vi "main.vi"() -> ()   [LabVIEW 2015]
uses:
  C:/Users/tosun_2/Desktop/Interop.TSMasterAPI.dll
panel:
  in  "停止":bool
  in  "close":bool
  out "log":string
  in  "main tab":enum32{"启动", "数据库", "收发界面"}(tab)
  in  "使能flexray通道数量":i32
  in  "LIN通道配置":T1(array[cluster]) {"AFunctionType" items=["T_MasterNode", "T_SlaveNode", "T_MonitorNode"]; "AProtocol" items=["LIN_PROTOCOL_13", "LIN_PROTOCOL_20", "LIN_PROTOCOL_21", "LIN_PROTOCOL_J2602"]; "FHWDeviceSubType" items=["TS_UNKNOWN_DEVICE"=0, "TC1001 "=3, "TL1001"=4, "TC1011"=5, "TC1002"=7, "TC1014"=8, "TC1026"=10, "TC1016"=11, "TC1012"=12, "TC1013 "=13, "TC1034"=15]; "FHWDeviceType" items=["BUS_UNKNOWN_TYPE", "TS_TCP_DEVICE", "XL_USB_DEVICE", "TS_USB_DEVICE", "PEAK_USB_DEVICE", "KVASER_USB_DEVICE", "RESERVED_DEVICE", "ICS_USB_DEVICE", "TS_TC1005_DEVICE"]; "FHWChannelIndex" items=["CHN1", "CHN2", "CHN3", "CHN4", "CHN5", "CHN6", "CHN7", "CHN8", "CHN9", "CHN10", "CHN11", "CHN12", "CHN13", "CHN14", "CHN15", "CHN16", "CHN17", "CHN18", "CHN19", "CHN20", "CHN21", "CHN22", "CHN23", "CHN24", "CHN25", "CHN26", "CHN27", "CHN28", "CHN29", "CHN30", "CHN31", "CHN32"]}
  in  "connect":bool
  in  "open":bool
  in  "TSMaster工程路径（可选）":path
  in  "使能CAN通道数量":i32
  in  "dbc路径":path
  in  "CAN通道配置":T2(array[cluster]) {"FHWDeviceSubType" items=["TS_UNKNOWN_DEVICE"=0, "TC1001 "=3, "TL1001"=4, "TC1011"=5, "TC1002"=7, "TC1014"=8, "TC1026"=10, "TC1016"=11, "TC1012"=12, "TC1013 "=13, "TC1034"=15]; "AControllerMode" items=["lfdmNormal", "lfdmACKOff", "lfdmRestricted"]; "AControllerType" items=["lfdtCAN", "lfdtISOFDCAN", "lfdtNonISOFDFDCAN"]; "FHWDeviceType" items=["BUS_UNKNOWN_TYPE", "TS_TCP_DEVICE", "XL_USB_DEVICE", "TS_USB_DEVICE", "PEAK_USB_DEVICE", "KVASER_USB_DEVICE", "RESERVED_DEVICE", "ICS_USB_DEVICE", "TS_TC1005_DEVICE"]; "FHWChannelIndex" items=["CHN1", "CHN2", "CHN3", "CHN4", "CHN5", "CHN6", "CHN7", "CHN8", "CHN9", "CHN10", "CHN11", "CHN12", "CHN13", "CHN14", "CHN15", "CHN16", "CHN17", "CHN18", "CHN19", "CHN20", "CHN21", "CHN22", "CHN23", "CHN24", "CHN25", "CHN26", "CHN27", "CHN28", "CHN29", "CHN30", "CHN31", "CHN32"]}
  in  "使能LIN通道数量":i32
  in  "ldf路径":path
  in  "xml路径":path
  in  "refresh databases":bool
  in  "数据库选项卡":enum32{"CAN", "LIN", "flexray"}(tab)
  out "CAN database":string(tree)="_1"
  out "LIN database":string(tree)="_1" caption="CAN database"
  out "flexray database":string(tree)="_1" caption="CAN database"
  in  "transmit":bool
  in  "transtab":enum32{"CAN", "LIN", "flexray"}(tab)
  in  "CAN通道":u8
  in  "CAN ID":i32 format="%x"
  in  "是否远程帧":bool
  in  "是否扩展帧":bool
  in  "是否CAN FD":bool
  in  "是否BRS":bool
  in  "DLC":u8
  in  "数据":u8[](array[numeric])
  in  "LIN通道":u8
  in  "LIN ID":u8 format="%x"
  in  "长度":u8
  in  "数据":u8[](array[numeric])
  in  "是否包含数据":bool=TRUE
  in  "数据 2":u8[](array[numeric])
  in  "flexray通道":u8
  in  "SlotId":u16
  in  "CycleNumber":u8
  in  "负载长度":u8
  in  "报文信息":i32(listbox)
  # "做主节点，不使能发送的flag时：设备将发送LIN报头，借此像从节点请求数据。做从节点时，仅更新数据，不会主动发送。"
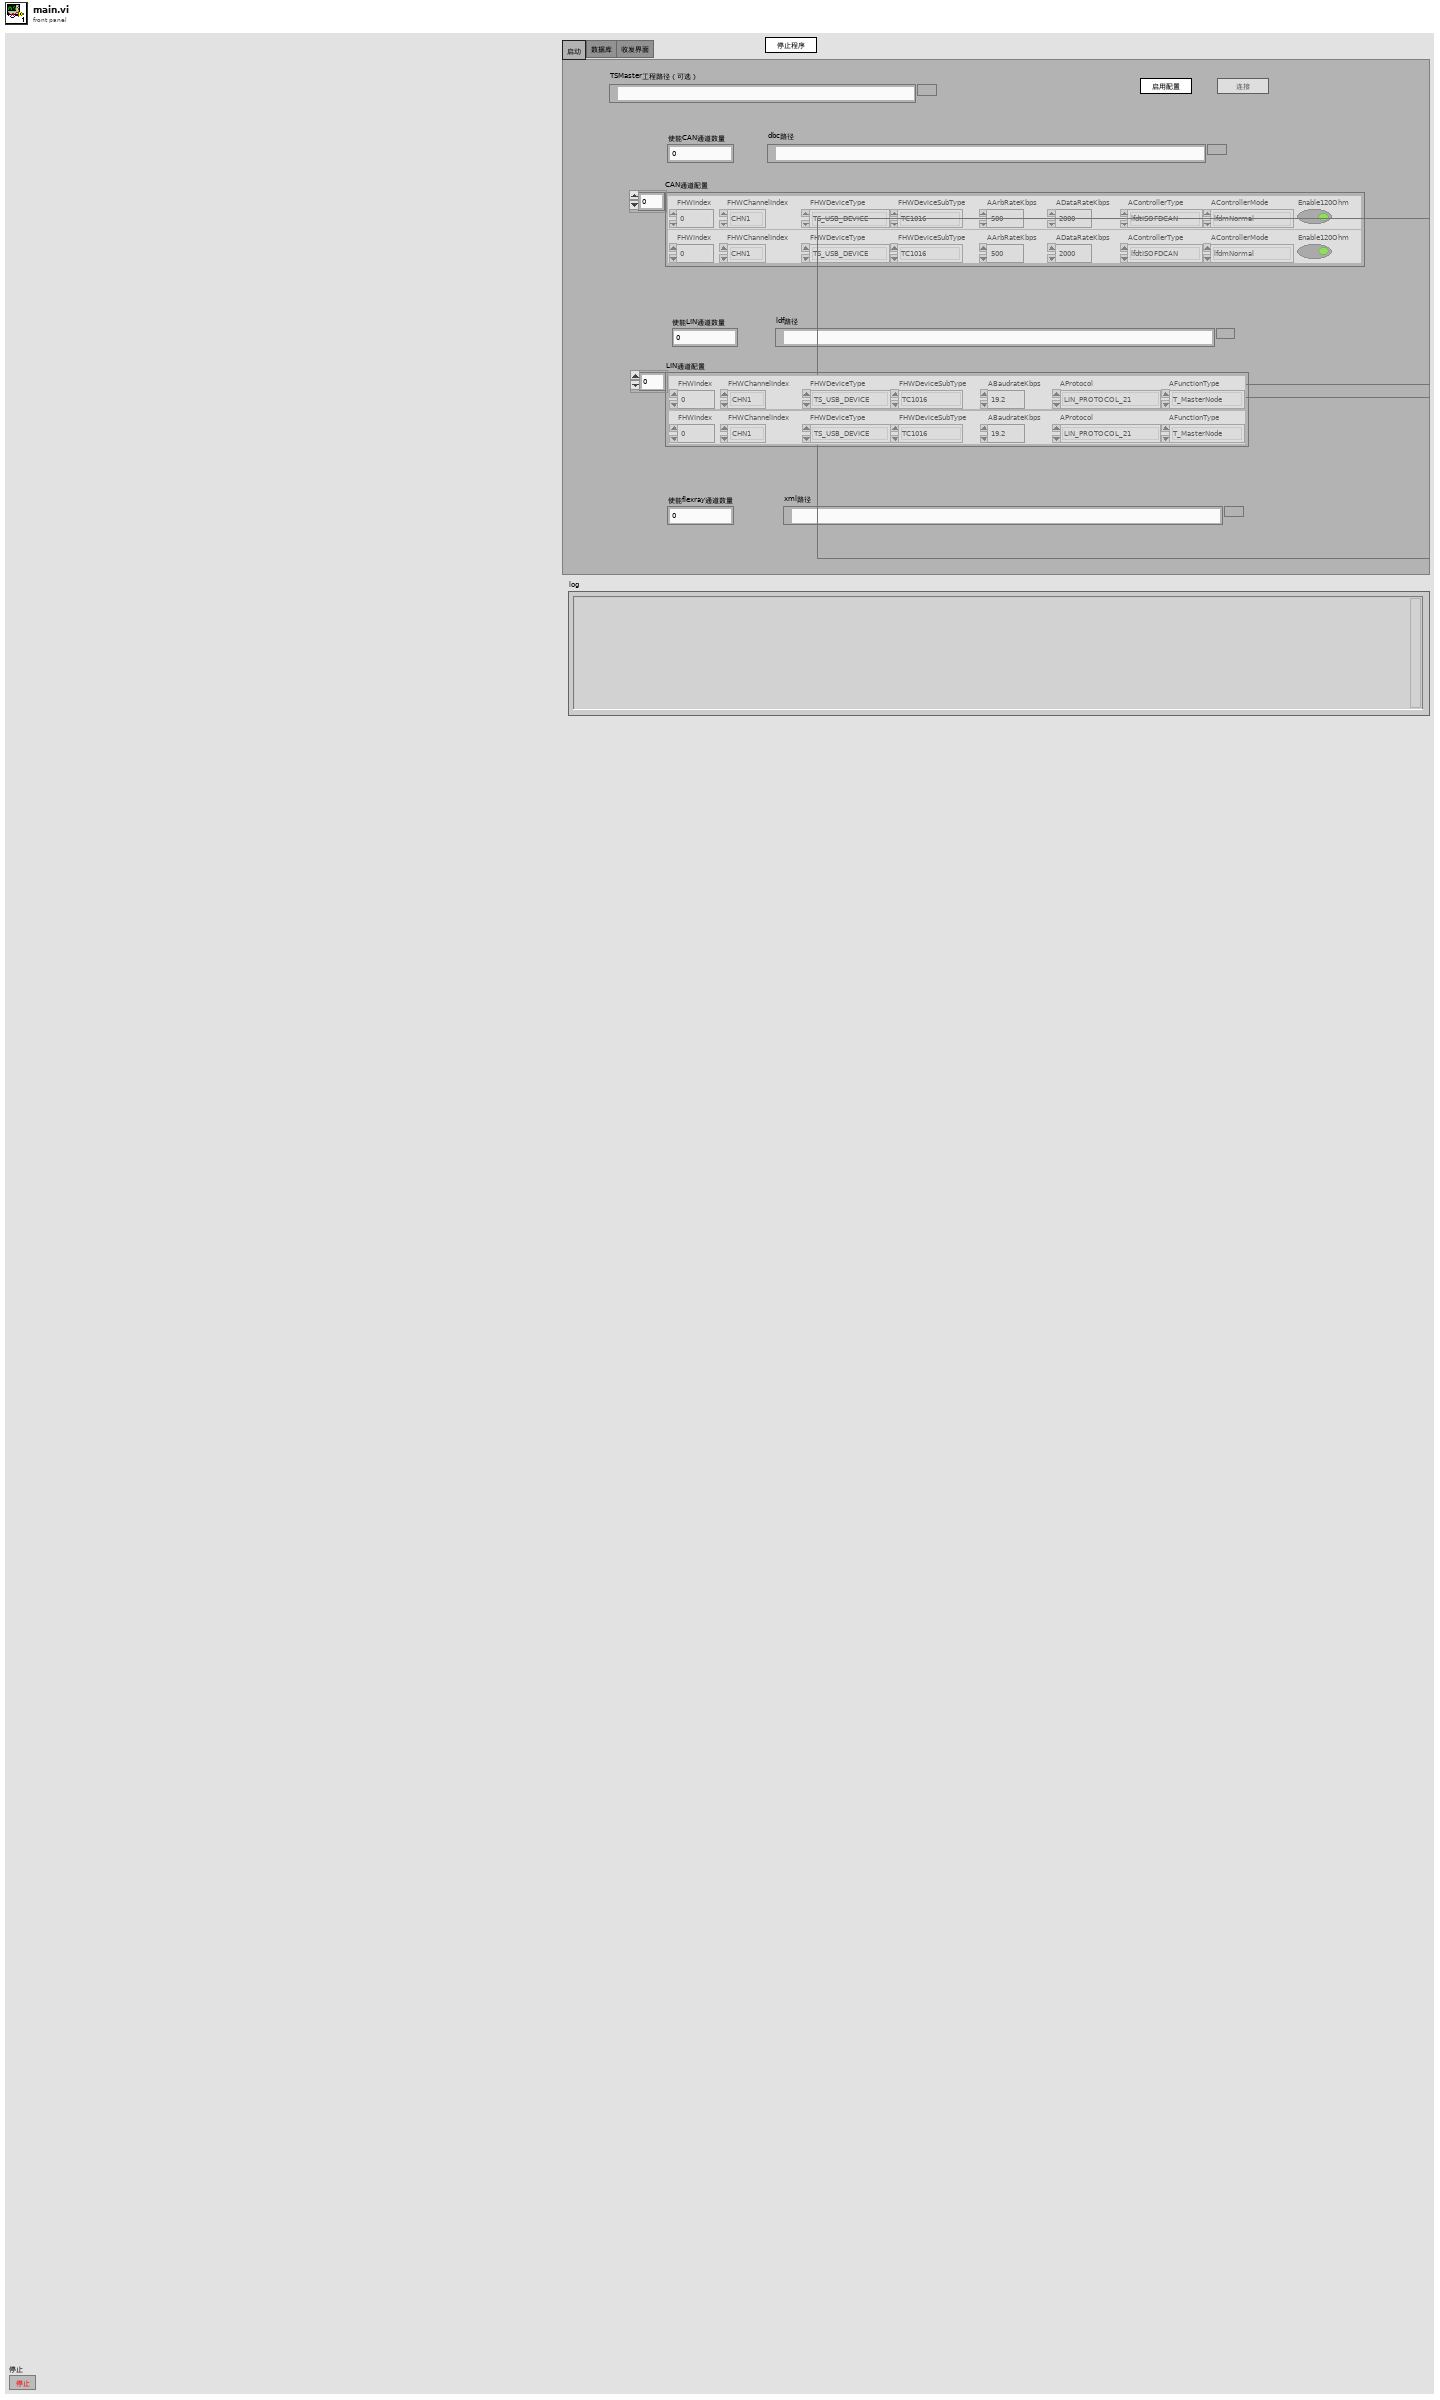
[diagram p1: front panel]
types:
  T1 = cluster{"FHWIndex":i32, "FHWChannelIndex":i32, "FHWDeviceType":i32, "FHWDeviceSubType":i32, "ABaudrateKbps":sgl, "AProtocol":i32, "AFunctionType":i32}[]
  T2 = cluster{"FHWIndex":i32, "FHWChannelIndex":i32, "FHWDeviceType":i32, "FHWDeviceSubType":i32, "AArbRateKbps":sgl, "ADataRateKbps":sgl, "AControllerType":i32, "AControllerMode":i32, "Enable120Ohm":bool}[]
  T3 = enum8{"Enabled", "Disabled", "Disabled and Grayed Out"}
  T4 = cluster{"Left Cell String":string, "Child Text":string[], "Child Tag":string, "Item Indent":i32, "Child Only?":bool, "Glyph Index":i32}[]
  T5 = cluster{"Left Cell String":string, "Child Text":string[], "Child Tag":string, "Item Indent":i32, "Child Only?":bool, "Glyph Index":i32}
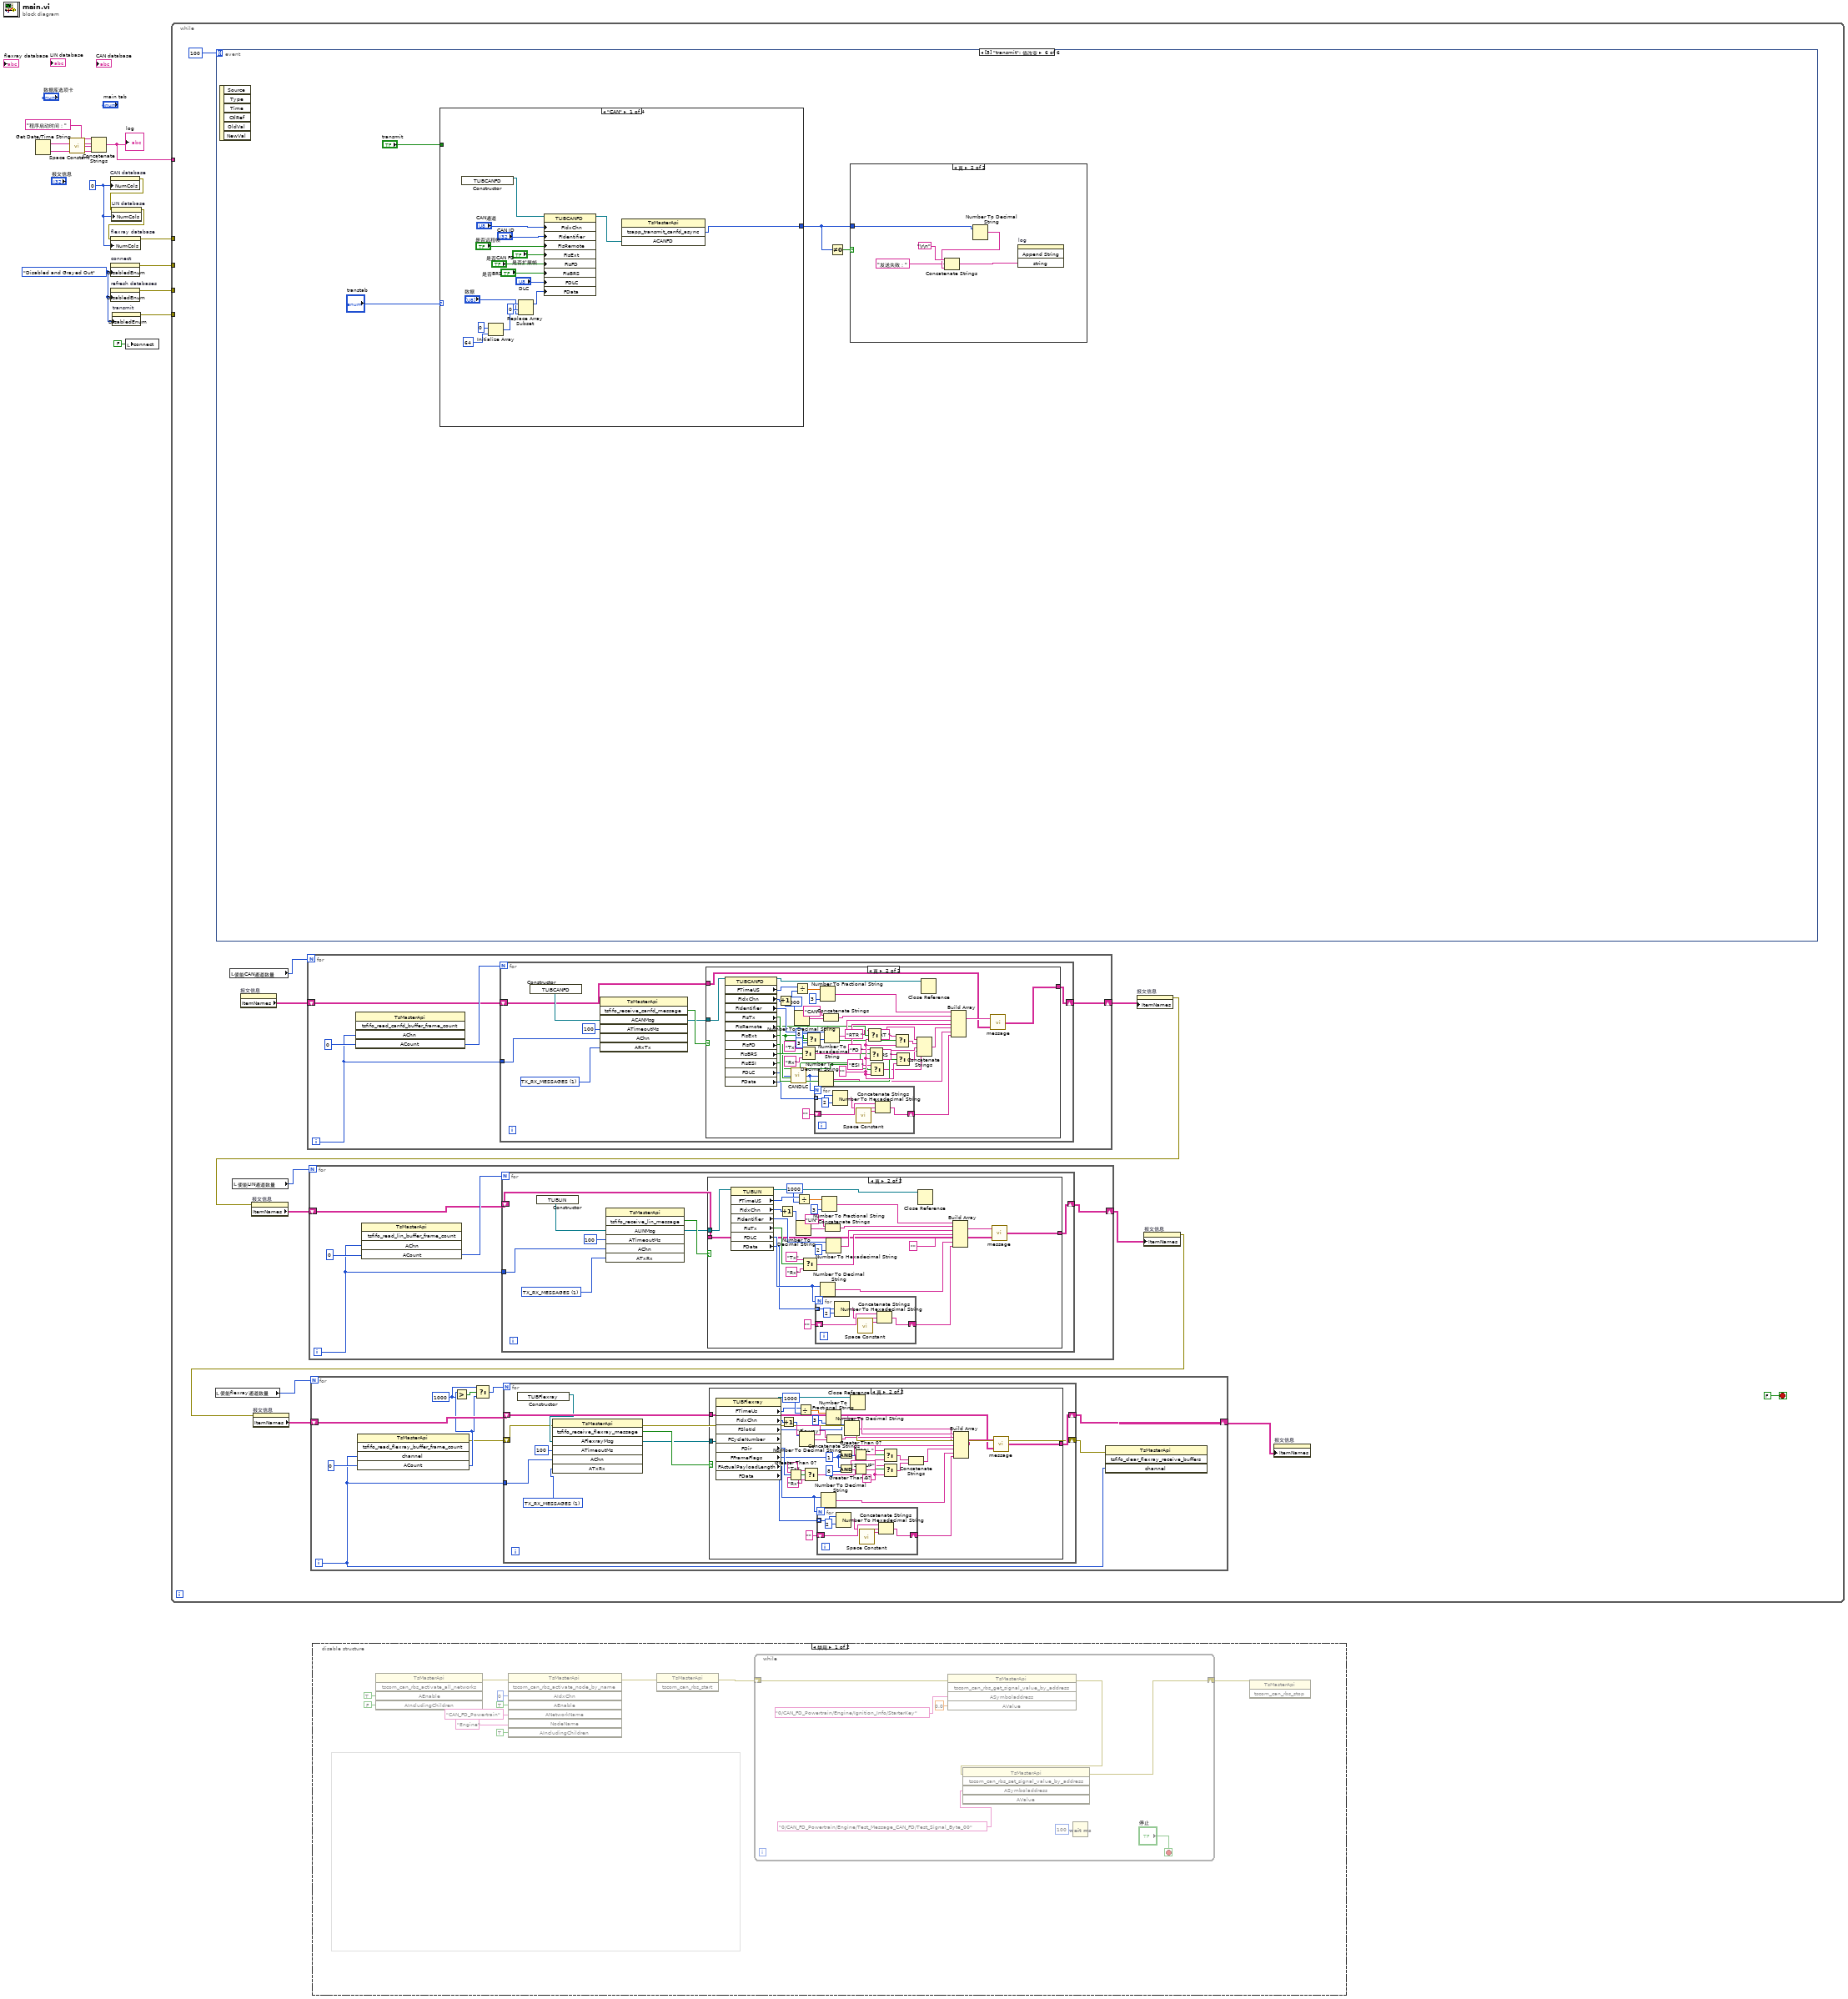
[diagram p0: block diagram]
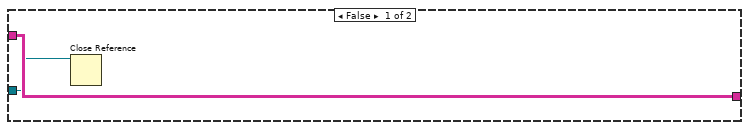
[diagram p3: hidden frame]
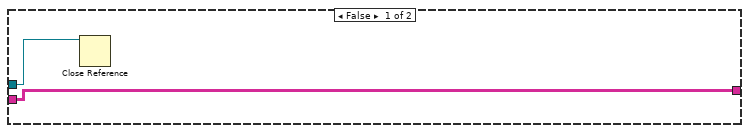
[diagram p4: hidden frame]
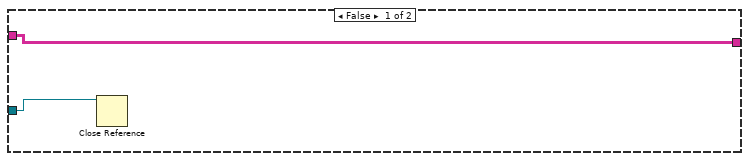
[diagram p5: hidden frame]
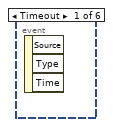
[diagram p6: hidden frame]
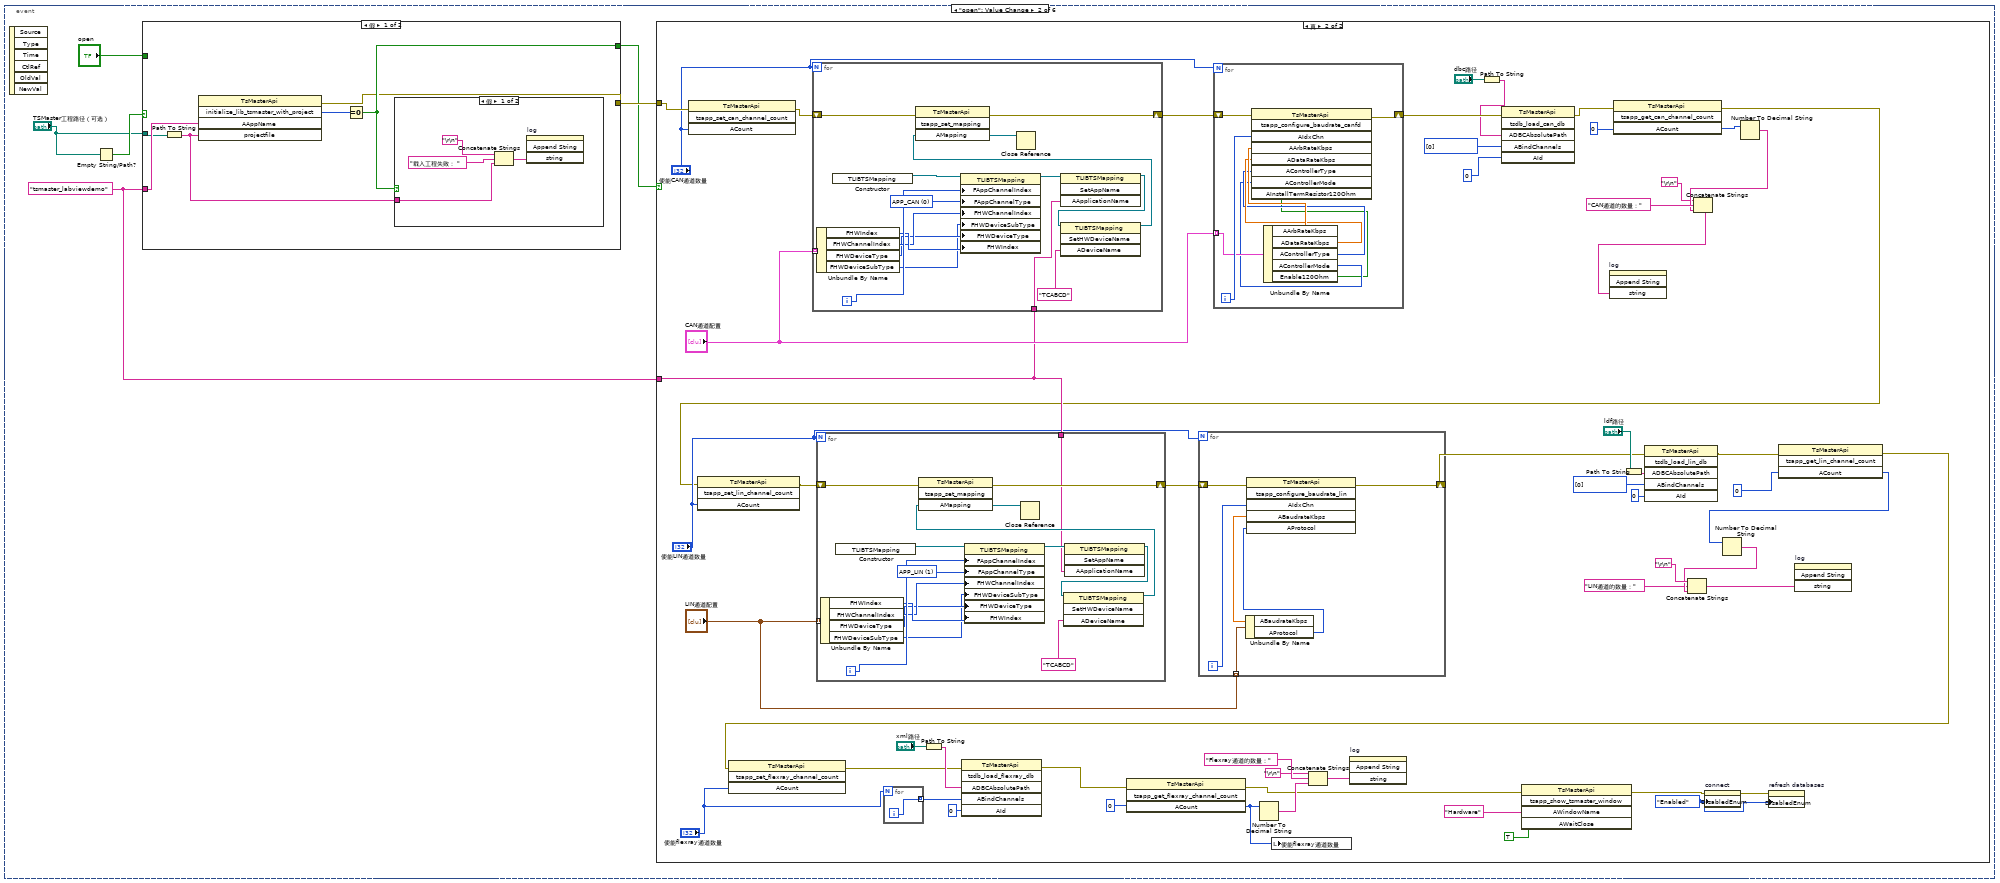
[diagram p7: hidden frame]
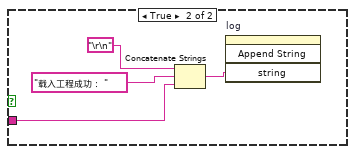
[diagram p9: hidden frame]
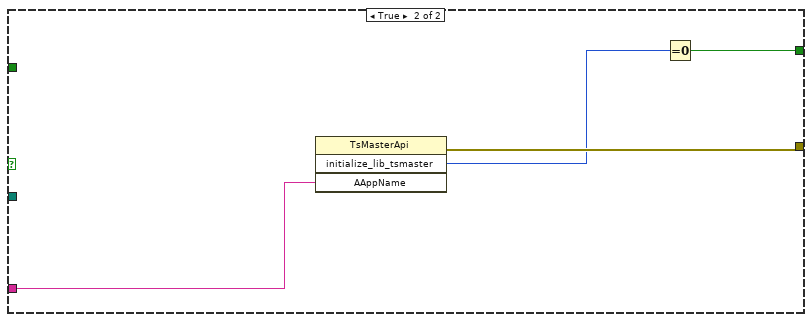
[diagram p10: hidden frame]
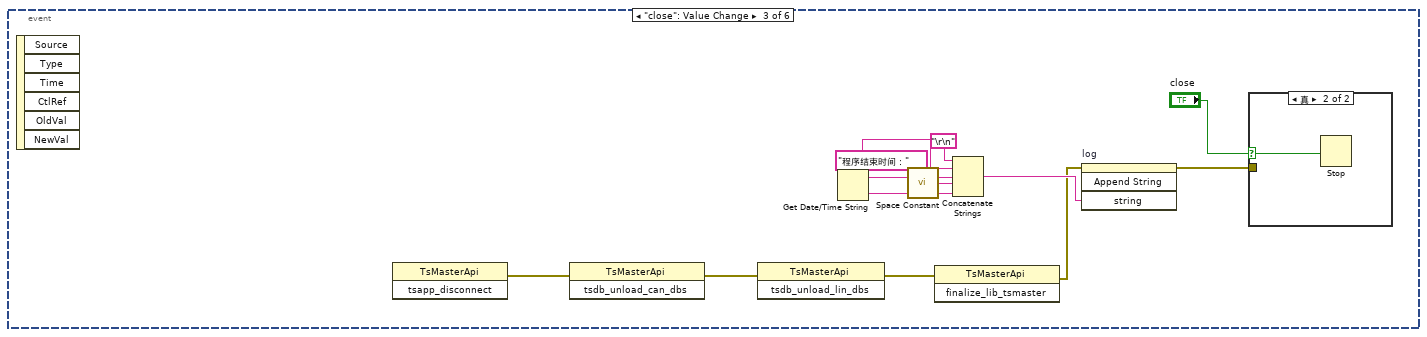
[diagram p11: hidden frame]
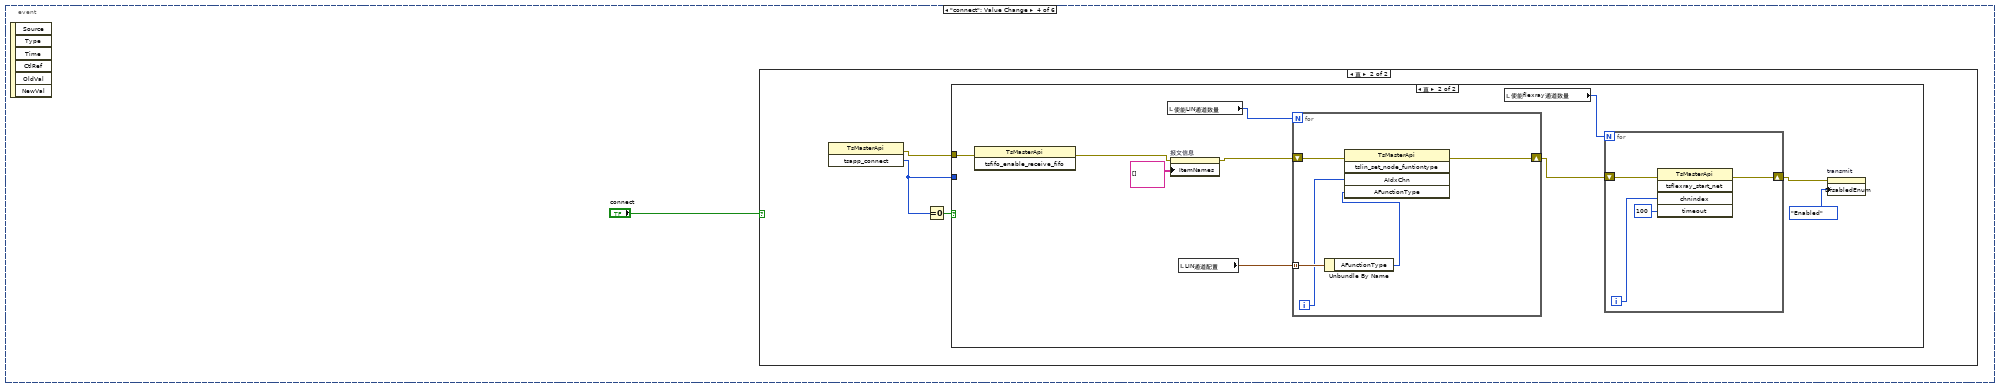
[diagram p13: hidden frame]
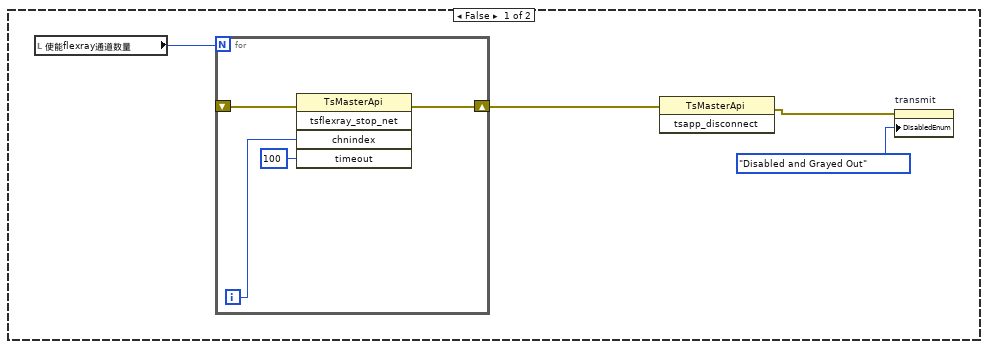
[diagram p14: hidden frame]
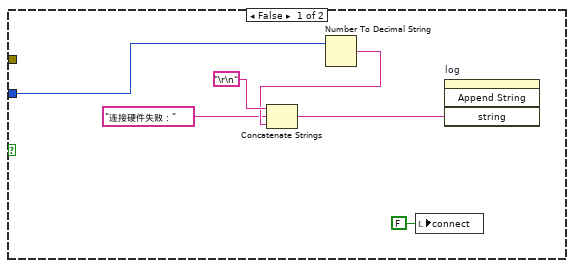
[diagram p15: hidden frame]
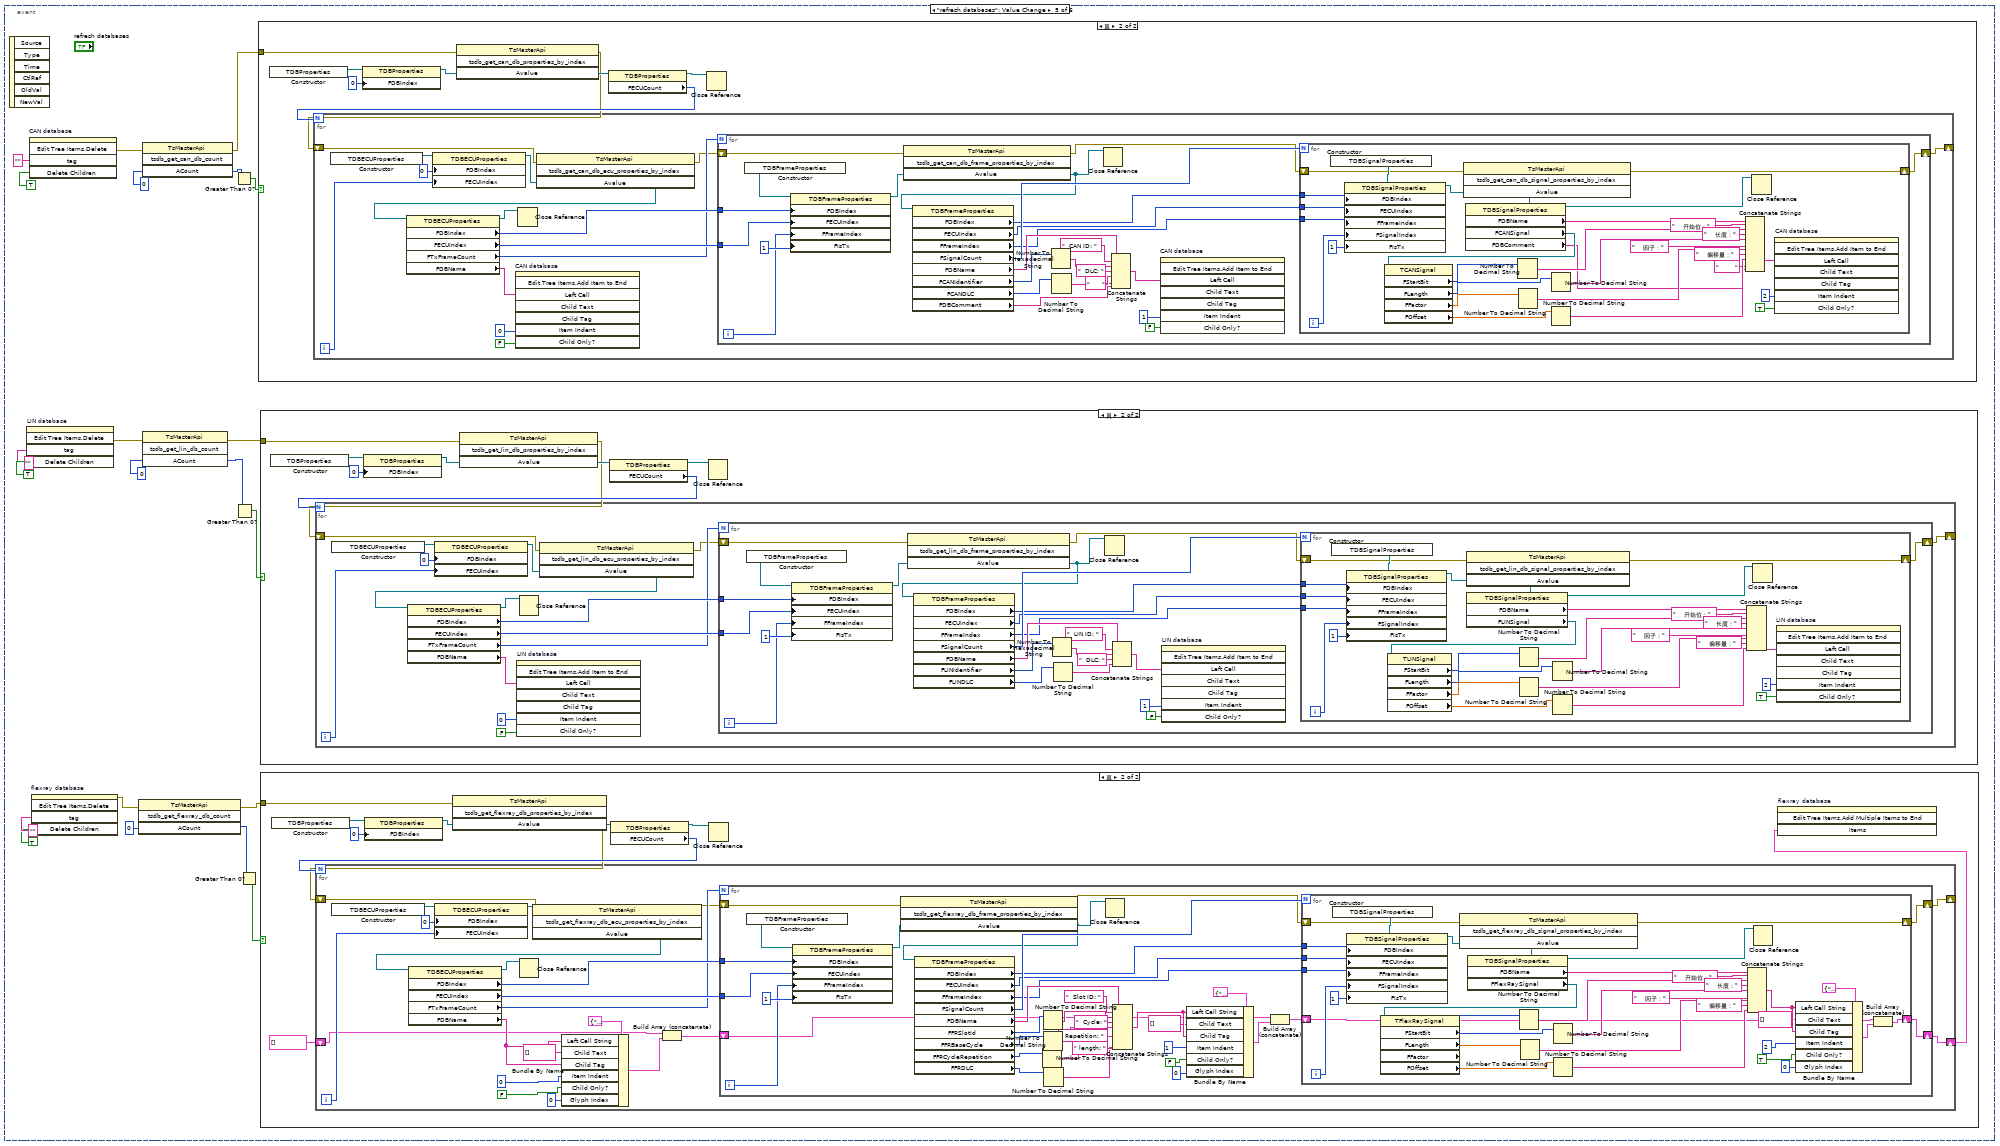
[diagram p16: hidden frame]
diagram:
  w3 = T3."Disabled and Grayed Out" ("禁用")
  w6 = u32 0 ("列数")
  n1 = Get Date/Time String() -> (date string=w13:string, time string=w12:string)  [unwired: 3 in]
  n2 = call <vilib>:"Space Constant.vi"() -> ("String"=w10:string)
  n3 = Concatenate Strings("程序启动时间：" ("字符串"), w13, w10, w12) -> (w11:string)
  "log" <- w11
  n4 = property on="CAN database" class="Tree (严格)"("NumCols"=w6) -> (error out=w9:errorcluster)  [unwired: 2 in, 1 out]
  n5 = property on="connect" class="Bool (严格)"("DisabledEnum"=w3) -> (error out=w5:errorcluster)  [unwired: 2 in, 1 out]
  n6 = property on="refresh databases" class="Bool"("DisabledEnum"=w3) -> (error out=w4:errorcluster)  [unwired: 2 in, 1 out]
  n7 = property on="LIN database" class="Tree (严格)"(error in=w9, "NumCols"=w6) -> (error out=w7:errorcluster)  [unwired: 1 in, 1 out]
  n8 = property on="flexray database" class="Tree (严格)"(error in=w7, "NumCols"=w6) -> (error out=w8:errorcluster)  [unwired: 1 in, 1 out]
  n9 = property on="transmit" class="Bool"("DisabledEnum"=w3) -> (error out=w2:errorcluster)  [unwired: 2 in, 1 out]
  n10 = local write "connect"(FALSE ("connect")) -> ()
  n11 = while {
    tunnel: w11 -> [_]
    tunnel: w8 -> [_]
    tunnel: w5 -> [_]
    tunnel: w4 -> [_]
    tunnel: w2 -> [_]
    stop <- FALSE stop-if-true
    n12 = local read "使能flexray通道数量"() -> (w17:i32)
    n13 = event shown="[5] \"transmit\": 值改变" {
      selector: _ -> [_ _ _ _ _ _]
      dyn-events: _ -> [_ _ _ _ _ _]
      timeout: 100 -> [_ _ _ _ _ _]
      event Timeout {
        n14 = event-data() -> ()  [unwired: 1 in, 3 out]
      }
      event "open": Value Change {
        w213 = "tsmaster_labviewdemo" ("AAppName")
        n15 = event-data() -> ()  [unwired: 1 in, 6 out]
        n16 = Empty String/Path?(string/path="TSMaster工程路径（可选）") -> (empty?=w218:bool)
        n17 = case shown="假" w218 {
          tunnel: "open" -> [_ _]
          tunnel: w213 -> [w327 w339]
          tunnel: "TSMaster工程路径（可选）" -> [w326 _]
          tunnel: [w324 w338] -> w214
          tunnel: [w322 w337] -> w215
          frame False {
            n18 = Path To String(path=w326) -> (string=w323:string)
            n19 = invoke on="调用节点" class="TsMasterApi" method="initialize_lib_tsmaster_with_project"("AAppName"=w327, "projectfile"=w323) -> (error out=w322:errorcluster, "initialize_lib_tsmaster_with_project"=w325:i32)  [unwired: 3 in, 3 out]
            n20 = Equal To 0?(x=w325) -> (x = 0?=w324:bool)
            n21 = case shown="假" w324 {
              tunnel: w323 -> [w329 w332]
              frame False {
                n22 = Concatenate Strings("\r\n", "载入工程失败： " ("字符串"), w329) -> (w328:string)
                n23 = invoke on="log" class="Str" method="Append String"("string"=w328) -> ()  [unwired: 3 in, 4 out]
              }
              frame True {
                n24 = Concatenate Strings("\r\n", "载入工程成功： " ("字符串"), w332) -> (w335:string)
                n25 = invoke on="log" class="Str" method="Append String"("string"=w335) -> ()  [unwired: 3 in, 4 out]
              }
            }
          }
          frame True {
            n26 = invoke on="调用节点" class="TsMasterApi" method="initialize_lib_tsmaster"("AAppName"=w339) -> (error out=w337:errorcluster, "initialize_lib_tsmaster"=w336:i32)  [unwired: 3 in, 2 out]
            n27 = Equal To 0?(x=w336) -> (x = 0?=w338:bool)
          }
        }
        n28 = case shown="真" w214 {
          tunnel: w215 -> [_ w261]
          tunnel: w213 -> [_ w256]
          frame False {
          }
          frame True {
            w221 = T3."Enabled" ("禁用")
            w250 = i32[] [0] items=["CHN1", "CHN2", "CHN3", "CHN4", "CHN5", "CHN6", "CHN7", "CHN8", "CHN9", "CHN10", "CHN11", "CHN12", "CHN13", "CHN14", "CHN15", "CHN16", "CHN17", "CHN18", "CHN19", "CHN20", "CHN21", "CHN22", "CHN23", "CHN24", "CHN25", "CHN26", "CHN27", "CHN28", "CHN29", "CHN30", "CHN31", "CHN32"] ("ABindChannels")
            w263 = i32[] [0] items=["CHN1", "CHN2", "CHN3", "CHN4", "CHN5", "CHN6", "CHN7", "CHN8", "CHN9", "CHN10", "CHN11", "CHN12", "CHN13", "CHN14", "CHN15", "CHN16", "CHN17", "CHN18", "CHN19", "CHN20", "CHN21", "CHN22", "CHN23", "CHN24", "CHN25", "CHN26", "CHN27", "CHN28", "CHN29", "CHN30", "CHN31", "CHN32"] ("ABindChannels")
            n29 = invoke on="调用节点" class="TsMasterApi" method="tsapp_set_can_channel_count"(error in=w261, "ACount"="使能CAN通道数量") -> (error out=w260:errorcluster)  [unwired: 2 in, 3 out]
            n30 = for {
              N: "使能CAN通道数量" -> [_]
              shift-right: [w321] -> w239
              shift-left: w260 -> [w314]
              tunnel: "CAN通道配置" -> [w318] mode=indexing
              tunnel: w256 -> [w308]
              i -> [w319]
              w320 = 0 items=["APP_CAN", "APP_LIN"] ("FAppChannelType")
              n31 = Unbundle By Name(w318) -> ("FHWIndex"=w317:i32, "FHWChannelIndex"=w316:i32, "FHWDeviceType"=w315:i32, "FHWDeviceSubType"=w306:i32)
              n32 = constructor class="TLIBTSMapping"() -> (reference out=w313:refnum<k24>)  [unwired: 3 in, 2 out]
              n33 = property on="属性节点" class="TLIBTSMapping"(reference=w313, "FAppChannelIndex"=w319, "FAppChannelType"=w320, "FHWChannelIndex"=w316, "FHWDeviceSubType"=w306, "FHWDeviceType"=w315, "FHWIndex"=w317) -> (reference out=w312:refnum<k24>)  [unwired: 1 in, 1 out]
              n34 = invoke on="调用节点" class="TLIBTSMapping" method="SetAppName"(reference=w312, "AApplicationName"=w308) -> (reference out=w310:refnum<k24>)  [unwired: 2 in, 3 out]
              n35 = invoke on="调用节点" class="TLIBTSMapping" method="SetHWDeviceName"(reference=w310, "ADeviceName"="TCABCD") -> (reference out=w309:refnum<k24>)  [unwired: 2 in, 3 out]
              n36 = invoke on="调用节点" class="TsMasterApi" method="tsapp_set_mapping"(error in=w314, "AMapping"=w309) -> (error out=w321:errorcluster, "AMapping"=w307:refnum<k24>)  [unwired: 2 in, 2 out]
              n37 = Close Reference(reference=w307) -> ()  [unwired: 1 in, 1 out]
            }
            n38 = for {
              N: "使能flexray通道数量" -> [_]
              tunnel: [w274] -> w224 mode=indexing
              i -> [w274]
            }
            n39 = Path To String(path="xml路径") -> (string=w227:string)
            n40 = for {
              N: "使能CAN通道数量" -> [_]
              shift-right: [w304] -> w266
              shift-left: w239 -> [w305]
              tunnel: "CAN通道配置" -> [w302] mode=indexing
              i -> [w303]
              n41 = Unbundle By Name(w302) -> ("AArbRateKbps"=w301:sgl, "ADataRateKbps"=w300:sgl, "AControllerType"=w299:i32, "AControllerMode"=w298:i32, "Enable120Ohm"=w297:bool)
              n42 = invoke on="调用节点" class="TsMasterApi" method="tsapp_configure_baudrate_canfd"(error in=w305, "AIdxChn"=w303, "AArbRateKbps"=w301, "ADataRateKbps"=w300, "AControllerType"=w299, "AControllerMode"=w298, "AInstallTermResistor120Ohm"=w297) -> (error out=w304:errorcluster)  [unwired: 2 in, 8 out]
            }
            n43 = Path To String(path="dbc路径") -> (string=w264:string)
            n44 = invoke on="调用节点" class="TsMasterApi" method="tsdb_load_can_db"(error in=w266, "ADBCAbsolutePath"=w264, "ABindChannels"=w263, "AId"=u32 0) -> (error out=w259:errorcluster)  [unwired: 2 in, 5 out]
            n45 = invoke on="调用节点" class="TsMasterApi" method="tsapp_get_can_channel_count"(error in=w259, "ACount"=0) -> (error out=w253:errorcluster, "ACount"=w268:i32)  [unwired: 2 in, 2 out]
            n46 = invoke on="调用节点" class="TsMasterApi" method="tsapp_set_lin_channel_count"(error in=w253, "ACount"="使能LIN通道数量") -> (error out=w257:errorcluster)  [unwired: 2 in, 3 out]
            n47 = for {
              N: "使能LIN通道数量" -> [_]
              shift-right: [w296] -> w240
              shift-left: w257 -> [w289]
              tunnel: "LIN通道配置" -> [w293] mode=indexing
              tunnel: w256 -> [w281]
              i -> [w294]
              w295 = 1 items=["APP_CAN", "APP_LIN"] ("FAppChannelType")
              n48 = Unbundle By Name(w293) -> ("FHWIndex"=w292:i32, "FHWChannelIndex"=w291:i32, "FHWDeviceType"=w290:i32, "FHWDeviceSubType"=w282:i32)
              n49 = constructor class="TLIBTSMapping"() -> (reference out=w288:refnum<k24>)  [unwired: 3 in, 2 out]
              n50 = property on="属性节点" class="TLIBTSMapping"(reference=w288, "FAppChannelIndex"=w294, "FAppChannelType"=w295, "FHWChannelIndex"=w291, "FHWDeviceSubType"=w282, "FHWDeviceType"=w290, "FHWIndex"=w292) -> (reference out=w287:refnum<k24>)  [unwired: 1 in, 1 out]
              n51 = invoke on="调用节点" class="TLIBTSMapping" method="SetAppName"(reference=w287, "AApplicationName"=w281) -> (reference out=w285:refnum<k24>)  [unwired: 2 in, 3 out]
              n52 = invoke on="调用节点" class="TLIBTSMapping" method="SetHWDeviceName"(reference=w285, "ADeviceName"="TCABCD") -> (reference out=w284:refnum<k24>)  [unwired: 2 in, 3 out]
              n53 = invoke on="调用节点" class="TsMasterApi" method="tsapp_set_mapping"(error in=w289, "AMapping"=w284) -> (error out=w296:errorcluster, "AMapping"=w283:refnum<k24>)  [unwired: 2 in, 2 out]
              n54 = Close Reference(reference=w283) -> ()  [unwired: 1 in, 1 out]
            }
            n55 = for {
              N: "使能LIN通道数量" -> [_]
              shift-right: [w275] -> w241
              shift-left: w240 -> [w280]
              tunnel: "LIN通道配置" -> [w279] mode=indexing
              i -> [w276]
              n56 = Unbundle By Name(w279) -> ("ABaudrateKbps"=w278:sgl, "AProtocol"=w277:i32)
              n57 = invoke on="调用节点" class="TsMasterApi" method="tsapp_configure_baudrate_lin"(error in=w280, "AIdxChn"=w276, "ABaudrateKbps"=w278, "AProtocol"=w277) -> (error out=w275:errorcluster)  [unwired: 2 in, 5 out]
            }
            n58 = Path To String(path="ldf路径") -> (string=w249:string)
            n59 = invoke on="调用节点" class="TsMasterApi" method="tsdb_load_lin_db"(error in=w241, "ADBCAbsolutePath"=w249, "ABindChannels"=w250, "AId"=u32 0) -> (error out=w252:errorcluster)  [unwired: 2 in, 5 out]
            n60 = Number To Decimal String(number=w268) -> (decimal integer string=w270:string)  [unwired: 1 in]
            n61 = Concatenate Strings("\r\n", "CAN通道的数量：" ("字符串"), w270) -> (w272:string)
            n62 = invoke on="log" class="Str" method="Append String"("string"=w272) -> ()  [unwired: 3 in, 4 out]
            n63 = invoke on="调用节点" class="TsMasterApi" method="tsapp_get_lin_channel_count"(error in=w252, "ACount"=0) -> (error out=w219:errorcluster, "ACount"=w247:i32)  [unwired: 2 in, 2 out]
            n64 = invoke on="调用节点" class="TsMasterApi" method="tsapp_set_flexray_channel_count"(error in=w219, "ACount"="使能flexray通道数量") -> (error out=w220:errorcluster)  [unwired: 2 in, 3 out]
            n65 = invoke on="调用节点" class="TsMasterApi" method="tsdb_load_flexray_db"(error in=w220, "ADBCAbsolutePath"=w227, "ABindChannels"=w224, "AId"=u32 0) -> (error out=w229:errorcluster)  [unwired: 2 in, 5 out]
            n66 = invoke on="调用节点" class="TsMasterApi" method="tsapp_get_flexray_channel_count"(error in=w229, "ACount"=0) -> (error out=w231:errorcluster, "ACount"=w230:i32)  [unwired: 2 in, 2 out]
            n67 = Number To Decimal String(number=w230) -> (decimal integer string=w233:string)  [unwired: 1 in]
            n68 = local write "使能flexray通道数量"(w230) -> ()
            n69 = Concatenate Strings("\r\n", "Flexray通道的数量：" ("字符串"), w233) -> (w235:string)
            n70 = invoke on="log" class="Str" method="Append String"("string"=w235) -> ()  [unwired: 3 in, 4 out]
            n71 = invoke on="调用节点" class="TsMasterApi" method="tsapp_show_tsmaster_window"(error in=w231, "AWindowName"="Hardware", "AWaitClose"=TRUE) -> (error out=w223:errorcluster)  [unwired: 2 in, 4 out]
            n72 = property on="connect" class="Bool (严格)"(error in=w223, "DisabledEnum"=w221) -> (error out=w222:errorcluster)  [unwired: 1 in, 1 out]
            n73 = Number To Decimal String(number=w247) -> (decimal integer string=w245:string)  [unwired: 1 in]
            n74 = Concatenate Strings("\r\n", "LIN通道的数量：" ("字符串"), w245) -> (w243:string)
            n75 = property on="refresh databases" class="Bool"(error in=w222, "DisabledEnum"=w221) -> ()  [unwired: 1 in, 2 out]
            n76 = invoke on="log" class="Str" method="Append String"("string"=w243) -> ()  [unwired: 3 in, 4 out]
          }
        }
      }
      event "close": Value Change {
        n77 = event-data() -> ()  [unwired: 1 in, 6 out]
        n78 = invoke on="调用节点" class="TsMasterApi" method="tsapp_disconnect"() -> (error out=w344:errorcluster)  [unwired: 3 in, 2 out]
        n79 = invoke on="调用节点" class="TsMasterApi" method="tsdb_unload_can_dbs"(error in=w344) -> (error out=w341:errorcluster)  [unwired: 2 in, 2 out]
        n80 = invoke on="调用节点" class="TsMasterApi" method="tsdb_unload_lin_dbs"(error in=w341) -> (error out=w340:errorcluster)  [unwired: 2 in, 2 out]
        n81 = Get Date/Time String() -> (date string=w350:string, time string=w349:string)  [unwired: 3 in]
        n82 = call <vilib>:"Space Constant.vi"() -> ("String"=w348:string)
        n83 = invoke on="调用节点" class="TsMasterApi" method="finalize_lib_tsmaster"(error in=w340) -> (error out=w343:errorcluster)  [unwired: 2 in, 2 out]
        n84 = Concatenate Strings("\r\n", "程序结束时间：" ("字符串"), w350, w348, w349) -> (w346:string)
        n85 = invoke on="log" class="Str" method="Append String"(error in=w343, "string"=w346) -> (error out=w342:errorcluster)  [unwired: 2 in, 3 out]
        n86 = case shown="真" "close" {
          selector: "close" -> [_ w352]
          tunnel: w342 -> [_ _]
          frame False {
          }
          frame True {
            n87 = Stop(stop? (T)=w352) -> ()
          }
        }
      }
      event "connect": Value Change {
        n88 = event-data() -> ()  [unwired: 1 in, 6 out]
        n89 = case shown="真" "connect" {
          frame False {
            n90 = local read "使能flexray通道数量"() -> (w357:i32)
            n91 = for {
              N: w357 -> [_]
              shift-right: [w360] -> w356
              shift-left: _ -> [w361]
              i -> [w359]
              n92 = invoke on="调用节点" class="TsMasterApi" method="tsflexray_stop_net"(error in=w361, "chnindex"=w359, "timeout"=100) -> (error out=w360:errorcluster)  [unwired: 2 in, 4 out]
            }
            n93 = invoke on="调用节点" class="TsMasterApi" method="tsapp_disconnect"(error in=w356) -> (error out=w354:errorcluster)  [unwired: 2 in, 2 out]
            n94 = property on="transmit" class="Bool"(error in=w354, "DisabledEnum"=T3."Disabled and Grayed Out" ("禁用")) -> ()  [unwired: 1 in, 2 out]
          }
          frame True {
            n95 = invoke on="调用节点" class="TsMasterApi" method="tsapp_connect"() -> (error out=w364:errorcluster, "tsapp_connect"=w362:i32)  [unwired: 3 in, 1 out]
            n96 = Equal To 0?(x=w362) -> (x = 0?=w363:bool)
            n97 = case shown="真" w363 {
              tunnel: w364 -> [_ w380]
              tunnel: w362 -> [w366 _]
              frame False {
                n98 = Number To Decimal String(number=w366) -> (decimal integer string=w369:string)  [unwired: 1 in]
                n99 = Concatenate Strings("\r\n", "连接硬件失败：" ("字符串"), w369) -> (w367:string)
                n100 = local write "connect"(FALSE ("connect")) -> ()
                n101 = invoke on="log" class="Str" method="Append String"("string"=w367) -> ()  [unwired: 3 in, 4 out]
              }
              frame True {
                n102 = invoke on="调用节点" class="TsMasterApi" method="tsfifo_enable_receive_fifo"(error in=w380) -> (error out=w378:errorcluster)  [unwired: 2 in, 2 out]
                n103 = local read "使能LIN通道数量"() -> (w377:i32)
                n104 = property on="报文信息" class="MCListbox (严格)"(error in=w378, "ItemNames"=string[][] [] ("项名")) -> (error out=w375:errorcluster)  [unwired: 1 in, 1 out]
                n105 = local read "LIN通道配置"() -> (w376:T1)
                n106 = for {
                  N: w377 -> [_]
                  tunnel: w376 -> [w389] mode=indexing
                  shift-right: [w385] -> w374
                  shift-left: w375 -> [w386]
                  i -> [w387]
                  n107 = Unbundle By Name(w389) -> ("AFunctionType"=w388:i32)
                  n108 = invoke on="调用节点" class="TsMasterApi" method="tslin_set_node_funtiontype"(error in=w386, "AIdxChn"=w387, "AFunctionType"=w388) -> (error out=w385:errorcluster)  [unwired: 2 in, 4 out]
                }
                n109 = local read "使能flexray通道数量"() -> (w373:i32)
                n110 = for {
                  N: w373 -> [_]
                  shift-right: [w383] -> w372
                  shift-left: w374 -> [w384]
                  i -> [w382]
                  n111 = invoke on="调用节点" class="TsMasterApi" method="tsflexray_start_net"(error in=w384, "chnindex"=w382, "timeout"=100) -> (error out=w383:errorcluster)  [unwired: 2 in, 4 out]
                }
                n112 = property on="transmit" class="Bool"(error in=w372, "DisabledEnum"=T3."Enabled" ("禁用")) -> ()  [unwired: 1 in, 2 out]
              }
            }
          }
        }
      }
      event "refresh databases": Value Change {
        n113 = event-data() -> ()  [unwired: 1 in, 6 out]
        n114 = invoke on="LIN database" class="Tree (严格)" method="Edit Tree Items.Delete"("tag"="" ("标识符"), "Delete Children"=TRUE ("删除子项？")) -> (error out=w401:errorcluster)  [unwired: 3 in, 4 out]
        n115 = invoke on="CAN database" class="Tree (严格)" method="Edit Tree Items.Delete"("tag"="" ("标识符"), "Delete Children"=TRUE ("删除子项？")) -> (error out=w406:errorcluster)  [unwired: 3 in, 4 out]
        n116 = invoke on="flexray database" class="Tree (严格)" method="Edit Tree Items.Delete"("tag"="" ("标识符"), "Delete Children"=TRUE ("删除子项？")) -> (error out=w390:errorcluster)  [unwired: 3 in, 4 out]
        n117 = invoke on="调用节点" class="TsMasterApi" method="tsdb_get_flexray_db_count"(error in=w390, "ACount"=0) -> (error out=w392:errorcluster, "ACount"=w395:i32)  [unwired: 2 in, 2 out]
        n118 = invoke on="调用节点" class="TsMasterApi" method="tsdb_get_can_db_count"(error in=w406, "ACount"=0) -> (error out=w407:errorcluster, "ACount"=w408:i32)  [unwired: 2 in, 2 out]
        n119 = invoke on="调用节点" class="TsMasterApi" method="tsdb_get_lin_db_count"(error in=w401, "ACount"=0) -> (error out=w398:errorcluster, "ACount"=w400:i32)  [unwired: 2 in, 2 out]
        n120 = Greater Than 0?(x=w408) -> (x > 0?=w409:bool)
        n121 = Greater Than 0?(x=w400) -> (x > 0?=w397:bool)
        n122 = Greater Than 0?(x=w395) -> (x > 0?=w391:bool)
        n123 = case shown="真" w409 {
          tunnel: w407 -> [_ w590]
          frame False {
          }
          frame True {
            n124 = constructor class="TDBProperties"() -> (reference out=w596:refnum<k24>)  [unwired: 3 in, 2 out]
            n125 = property on="属性节点" class="TDBProperties"(reference=w596, "FDBIndex"=0) -> (reference out=w594:refnum<k24>)  [unwired: 1 in, 1 out]
            n126 = invoke on="调用节点" class="TsMasterApi" method="tsdb_get_can_db_properties_by_index"(error in=w590, "Avalue"=w594) -> (error out=w589:errorcluster, "Avalue"=w593:refnum<k24>)  [unwired: 2 in, 2 out]
            n127 = property on="属性节点" class="TDBProperties"(reference=w593) -> (reference out=w591:refnum<k24>, "FECUCount"=w592:i32)  [unwired: 1 in, 1 out]
            n128 = for {
              N: w592 -> [_]
              shift-right: [w598] -> _
              shift-left: w589 -> [w607]
              i -> [w609]
              n129 = constructor class="TDBECUProperties"() -> (reference out=w611:refnum<k24>)  [unwired: 3 in, 2 out]
              n130 = property on="属性节点" class="TDBECUProperties"(reference=w611, "FDBIndex"=0, "FECUIndex"=w609) -> (reference out=w608:refnum<k24>)  [unwired: 1 in, 1 out]
              n131 = invoke on="调用节点" class="TsMasterApi" method="tsdb_get_can_db_ecu_properties_by_index"(error in=w607, "Avalue"=w608) -> (error out=w599:errorcluster, "Avalue"=w606:refnum<k24>)  [unwired: 2 in, 2 out]
              n132 = property on="属性节点" class="TDBECUProperties"(reference=w606) -> (reference out=w600:refnum<k24>, "FDBIndex"=w603:i32, "FECUIndex"=w602:i32, "FTxFrameCount"=w601:i32, "FDBName"=w604:string)  [unwired: 1 in, 1 out]
              n133 = invoke on="CAN database" class="Tree (严格)" method="Edit Tree Items.Add Item to End"("Left Cell"=w604, "Item Indent"=0 ("新项缩进"), "Child Only?"=FALSE ("仅作为子项？")) -> ()  [unwired: 5 in, 8 out]
              n134 = Close Reference(reference=w600) -> ()  [unwired: 1 in, 1 out]
              n135 = for {
                N: w601 -> [_]
                tunnel: w603 -> [w636]
                tunnel: w602 -> [w635]
                shift-right: [w613] -> w598
                shift-left: w599 -> [w632]
                i -> [w633]
                n136 = constructor class="TDBFrameProperties"() -> (reference out=w637:refnum<k24>)  [unwired: 3 in, 2 out]
                n137 = property on="属性节点" class="TDBFrameProperties"(reference=w637, "FDBIndex"=w636, "FECUIndex"=w635, "FFrameIndex"=w633, "FIsTx"=u8 1) -> (reference out=w631:refnum<k24>)  [unwired: 1 in, 1 out]
                n138 = invoke on="调用节点" class="TsMasterApi" method="tsdb_get_can_db_frame_properties_by_index"(error in=w632, "Avalue"=w631) -> (error out=w614:errorcluster, "Avalue"=w618:refnum<k24>)  [unwired: 2 in, 2 out]
                n139 = property on="属性节点" class="TDBFrameProperties"(reference=w618) -> ("FDBIndex"=w617:i32, "FECUIndex"=w616:i32, "FFrameIndex"=w615:i32, "FSignalCount"=w619:i32, "FDBName"=w630:string, "FCANIdentifier"=w627:i32, "FCANDLC"=w623:i32, "FDBComment"=w620:string)  [unwired: 1 in, 2 out]
                n140 = Number To Hexadecimal String(2:w627) -> (0:w626:string)  [unwired: 1 in]
                n141 = Number To Decimal String(number=w623) -> (decimal integer string=w622:string)  [unwired: 1 in]
                n142 = Close Reference(reference=w618) -> ()  [unwired: 1 in, 1 out]
                n143 = Concatenate Strings(w630, "  CAN ID: " ("字符串"), w626, "  DLC: " ("字符串"), w622, "      " ("字符串"), w620) -> (w629:string)
                n144 = invoke on="CAN database" class="Tree (严格)" method="Edit Tree Items.Add Item to End"("Left Cell"=w629, "Item Indent"=1 ("新项缩进"), "Child Only?"=FALSE ("仅作为子项？")) -> ()  [unwired: 5 in, 8 out]
                n145 = for {
                  N: w619 -> [_]
                  tunnel: w617 -> [w664]
                  tunnel: w616 -> [w663]
                  tunnel: w615 -> [w662]
                  shift-right: [w658] -> w613
                  shift-left: w614 -> [w661]
                  i -> [w665]
                  n146 = constructor class="TDBSignalProperties"() -> (reference out=w667:refnum<k24>)  [unwired: 3 in, 2 out]
                  n147 = property on="属性节点" class="TDBSignalProperties"(reference=w667, "FDBIndex"=w664, "FECUIndex"=w663, "FFrameIndex"=w662, "FSignalIndex"=w665, "FIsTx"=u8 1) -> (reference out=w660:refnum<k24>)  [unwired: 1 in, 1 out]
                  n148 = invoke on="调用节点" class="TsMasterApi" method="tsdb_get_can_db_signal_properties_by_index"(error in=w661, "Avalue"=w660) -> (error out=w658:errorcluster, "Avalue"=w659:refnum<k24>)  [unwired: 2 in, 2 out]
                  n149 = property on="属性节点" class="TDBSignalProperties"(reference=w659) -> (reference out=w657:refnum<k24>, "FDBName"=w653:string, "FCANSignal"=w656:refnum<k24>, "FDBComment"=w639:string)  [unwired: 1 in, 1 out]
                  n150 = property on="属性节点" class="TCANSignal"(reference=w656) -> ("FStartBit"=w648:i32, "FLength"=w649:i32, "FFactor"=w650:dbl, "FOffset"=w651:dbl)  [unwired: 1 in, 2 out]
                  n151 = Number To Decimal String(number=w648) -> (decimal integer string=w647:string)  [unwired: 1 in]
                  n152 = Number To Decimal String(number=w650) -> (decimal integer string=w643:string)  [unwired: 1 in]
                  n153 = Number To Decimal String(number=w649) -> (decimal integer string=w645:string)  [unwired: 1 in]
                  n154 = Number To Decimal String(number=w651) -> (decimal integer string=w641:string)  [unwired: 1 in]
                  n155 = Concatenate Strings(w653, "    开始位：" ("字符串"), w647, "    长度：" ("字符串"), w645, "    因子：" ("字符串"), w643, "    偏移量：" ("字符串"), w641, "        " ("字符串"), w639) -> (w654:string)
                  n156 = Close Reference(reference=w657) -> ()  [unwired: 1 in, 1 out]
                  n157 = invoke on="CAN database" class="Tree (严格)" method="Edit Tree Items.Add Item to End"("Left Cell"=w654, "Item Indent"=2 ("新项缩进"), "Child Only?"=TRUE ("仅作为子项？")) -> ()  [unwired: 5 in, 8 out]
                }
              }
            }
            n158 = Close Reference(reference=w591) -> ()  [unwired: 1 in, 1 out]
          }
        }
        n159 = case shown="真" w397 {
          tunnel: w398 -> [_ w515]
          frame False {
          }
          frame True {
            n160 = constructor class="TDBProperties"() -> (reference out=w521:refnum<k24>)  [unwired: 3 in, 2 out]
            n161 = property on="属性节点" class="TDBProperties"(reference=w521, "FDBIndex"=0) -> (reference out=w519:refnum<k24>)  [unwired: 1 in, 1 out]
            n162 = invoke on="调用节点" class="TsMasterApi" method="tsdb_get_lin_db_properties_by_index"(error in=w515, "Avalue"=w519) -> (error out=w514:errorcluster, "Avalue"=w518:refnum<k24>)  [unwired: 2 in, 2 out]
            n163 = property on="属性节点" class="TDBProperties"(reference=w518) -> (reference out=w516:refnum<k24>, "FECUCount"=w517:i32)  [unwired: 1 in, 1 out]
            n164 = for {
              N: w517 -> [_]
              shift-right: [w523] -> _
              shift-left: w514 -> [w532]
              i -> [w534]
              n165 = constructor class="TDBECUProperties"() -> (reference out=w536:refnum<k24>)  [unwired: 3 in, 2 out]
              n166 = property on="属性节点" class="TDBECUProperties"(reference=w536, "FDBIndex"=0, "FECUIndex"=w534) -> (reference out=w533:refnum<k24>)  [unwired: 1 in, 1 out]
              n167 = invoke on="调用节点" class="TsMasterApi" method="tsdb_get_lin_db_ecu_properties_by_index"(error in=w532, "Avalue"=w533) -> (error out=w524:errorcluster, "Avalue"=w531:refnum<k24>)  [unwired: 2 in, 2 out]
              n168 = property on="属性节点" class="TDBECUProperties"(reference=w531) -> (reference out=w525:refnum<k24>, "FDBIndex"=w528:i32, "FECUIndex"=w527:i32, "FTxFrameCount"=w526:i32, "FDBName"=w529:string)  [unwired: 1 in, 1 out]
              n169 = invoke on="LIN database" class="Tree (严格)" method="Edit Tree Items.Add Item to End"("Left Cell"=w529, "Item Indent"=0 ("新项缩进"), "Child Only?"=FALSE ("仅作为子项？")) -> ()  [unwired: 5 in, 8 out]
              n170 = Close Reference(reference=w525) -> ()  [unwired: 1 in, 1 out]
              n171 = for {
                N: w526 -> [_]
                tunnel: w528 -> [w559]
                tunnel: w527 -> [w558]
                shift-right: [w538] -> w523
                shift-left: w524 -> [w555]
                i -> [w556]
                n172 = constructor class="TDBFrameProperties"() -> (reference out=w560:refnum<k24>)  [unwired: 3 in, 2 out]
                n173 = property on="属性节点" class="TDBFrameProperties"(reference=w560, "FDBIndex"=w559, "FECUIndex"=w558, "FFrameIndex"=w556, "FIsTx"=u8 1) -> (reference out=w554:refnum<k24>)  [unwired: 1 in, 1 out]
                n174 = invoke on="调用节点" class="TsMasterApi" method="tsdb_get_lin_db_frame_properties_by_index"(error in=w555, "Avalue"=w554) -> (error out=w539:errorcluster, "Avalue"=w543:refnum<k24>)  [unwired: 2 in, 2 out]
                n175 = property on="属性节点" class="TDBFrameProperties"(reference=w543) -> ("FDBIndex"=w542:i32, "FECUIndex"=w541:i32, "FFrameIndex"=w540:i32, "FSignalCount"=w544:i32, "FDBName"=w553:string, "FLINIdentifier"=w550:i32, "FLINDLC"=w546:i32)  [unwired: 1 in, 2 out]
                n176 = Number To Hexadecimal String(2:w550) -> (0:w549:string)  [unwired: 1 in]
                n177 = Number To Decimal String(number=w546) -> (decimal integer string=w545:string)  [unwired: 1 in]
                n178 = Close Reference(reference=w543) -> ()  [unwired: 1 in, 1 out]
                n179 = Concatenate Strings(w553, "  LIN ID: " ("字符串"), w549, "  DLC: " ("字符串"), w545) -> (w552:string)
                n180 = invoke on="LIN database" class="Tree (严格)" method="Edit Tree Items.Add Item to End"("Left Cell"=w552, "Item Indent"=1 ("新项缩进"), "Child Only?"=FALSE ("仅作为子项？")) -> ()  [unwired: 5 in, 8 out]
                n181 = for {
                  N: w544 -> [_]
                  tunnel: w542 -> [w585]
                  tunnel: w541 -> [w584]
                  tunnel: w540 -> [w583]
                  shift-right: [w579] -> w538
                  shift-left: w539 -> [w582]
                  i -> [w586]
                  n182 = constructor class="TDBSignalProperties"() -> (reference out=w588:refnum<k24>)  [unwired: 3 in, 2 out]
                  n183 = property on="属性节点" class="TDBSignalProperties"(reference=w588, "FDBIndex"=w585, "FECUIndex"=w584, "FFrameIndex"=w583, "FSignalIndex"=w586, "FIsTx"=u8 1) -> (reference out=w581:refnum<k24>)  [unwired: 1 in, 1 out]
                  n184 = invoke on="调用节点" class="TsMasterApi" method="tsdb_get_lin_db_signal_properties_by_index"(error in=w582, "Avalue"=w581) -> (error out=w579:errorcluster, "Avalue"=w580:refnum<k24>)  [unwired: 2 in, 2 out]
                  n185 = property on="属性节点" class="TDBSignalProperties"(reference=w580) -> (reference out=w578:refnum<k24>, "FDBName"=w574:string, "FLINSignal"=w577:refnum<k24>)  [unwired: 1 in, 1 out]
                  n186 = property on="属性节点" class="TLINSignal"(reference=w577) -> ("FStartBit"=w569:i32, "FLength"=w570:i32, "FFactor"=w571:dbl, "FOffset"=w572:dbl)  [unwired: 1 in, 2 out]
                  n187 = Number To Decimal String(number=w569) -> (decimal integer string=w568:string)  [unwired: 1 in]
                  n188 = Number To Decimal String(number=w571) -> (decimal integer string=w564:string)  [unwired: 1 in]
                  n189 = Number To Decimal String(number=w570) -> (decimal integer string=w566:string)  [unwired: 1 in]
                  n190 = Number To Decimal String(number=w572) -> (decimal integer string=w562:string)  [unwired: 1 in]
                  n191 = Concatenate Strings(w574, "    开始位：" ("字符串"), w568, "    长度：" ("字符串"), w566, "    因子：" ("字符串"), w564, "    偏移量：" ("字符串"), w562) -> (w575:string)
                  n192 = Close Reference(reference=w578) -> ()  [unwired: 1 in, 1 out]
                  n193 = invoke on="LIN database" class="Tree (严格)" method="Edit Tree Items.Add Item to End"("Left Cell"=w575, "Item Indent"=2 ("新项缩进"), "Child Only?"=TRUE ("仅作为子项？")) -> ()  [unwired: 5 in, 8 out]
                }
              }
            }
            n194 = Close Reference(reference=w516) -> ()  [unwired: 1 in, 1 out]
          }
        }
        n195 = case shown="真" w391 {
          tunnel: w392 -> [_ w414]
          frame False {
          }
          frame True {
            n196 = constructor class="TDBProperties"() -> (reference out=w420:refnum<k24>)  [unwired: 3 in, 2 out]
            n197 = property on="属性节点" class="TDBProperties"(reference=w420, "FDBIndex"=0) -> (reference out=w418:refnum<k24>)  [unwired: 1 in, 1 out]
            n198 = invoke on="调用节点" class="TsMasterApi" method="tsdb_get_flexray_db_properties_by_index"(error in=w414, "Avalue"=w418) -> (error out=w413:errorcluster, "Avalue"=w417:refnum<k24>)  [unwired: 2 in, 2 out]
            n199 = property on="属性节点" class="TDBProperties"(reference=w417) -> (reference out=w415:refnum<k24>, "FECUCount"=w416:i32)  [unwired: 1 in, 1 out]
            n200 = for {
              N: w416 -> [_]
              shift-right: [w431] -> _
              shift-left: w413 -> [w438]
              shift-right: [w421] -> w411
              shift-left: T4 [] ("多项") -> [w424]
              i -> [w440]
              n201 = constructor class="TDBECUProperties"() -> (reference out=w442:refnum<k24>)  [unwired: 3 in, 2 out]
              n202 = property on="属性节点" class="TDBECUProperties"(reference=w442, "FDBIndex"=0, "FECUIndex"=w440) -> (reference out=w439:refnum<k24>)  [unwired: 1 in, 1 out]
              n203 = invoke on="调用节点" class="TsMasterApi" method="tsdb_get_flexray_db_ecu_properties_by_index"(error in=w438, "Avalue"=w439) -> (error out=w432:errorcluster, "Avalue"=w437:refnum<k24>)  [unwired: 2 in, 2 out]
              n204 = property on="属性节点" class="TDBECUProperties"(reference=w437) -> (reference out=w433:refnum<k24>, "FDBIndex"=w436:i32, "FECUIndex"=w435:i32, "FTxFrameCount"=w434:i32, "FDBName"=w428:string)  [unwired: 1 in, 1 out]
              n205 = Close Reference(reference=w433) -> ()  [unwired: 1 in, 1 out]
              n206 = Bundle By Name(cluster=T5 {"Left Cell String"="", "Child Text"=[], "Child Tag"="", "Item Indent"=0, "Child Only?"=FALSE, "Glyph Index"=0} ("Item"), "Left Cell String"=w428, "Child Text"=string[] [], "Child Tag"=w428, "Item Indent"=0 ("新项缩进"), "Child Only?"=FALSE ("仅作为子项？"), "Glyph Index"=0) -> (w423:T5)
              n207 = Build Array (concatenate)(w424, w423) -> (w422:T4)
              n208 = for {
                N: w434 -> [_]
                tunnel: w436 -> [w478]
                tunnel: w435 -> [w477]
                shift-right: [w463] -> w431
                shift-left: w432 -> [w474]
                shift-right: [w443] -> w421
                shift-left: w422 -> [w444]
                i -> [w475]
                n209 = constructor class="TDBFrameProperties"() -> (reference out=w479:refnum<k24>)  [unwired: 3 in, 2 out]
                n210 = property on="属性节点" class="TDBFrameProperties"(reference=w479, "FDBIndex"=w478, "FECUIndex"=w477, "FFrameIndex"=w475, "FIsTx"=u8 1) -> (reference out=w473:refnum<k24>)  [unwired: 1 in, 1 out]
                n211 = invoke on="调用节点" class="TsMasterApi" method="tsdb_get_flexray_db_frame_properties_by_index"(error in=w474, "Avalue"=w473) -> (error out=w464:errorcluster, "Avalue"=w468:refnum<k24>)  [unwired: 2 in, 2 out]
                n212 = property on="属性节点" class="TDBFrameProperties"(reference=w468) -> ("FDBIndex"=w467:i32, "FECUIndex"=w466:i32, "FFrameIndex"=w465:i32, "FSignalCount"=w469:i32, "FDBName"=w472:string, "FFRSlotId"=w462:i16, "FFRBaseCycle"=w460:u8, "FFRCycleRepetition"=w457:u8, "FFRDLC"=w456:i16)  [unwired: 1 in, 2 out]
                n213 = Number To Decimal String(number=w457) -> (decimal integer string=w455:string)  [unwired: 1 in]
                n214 = Number To Decimal String(number=w462) -> (decimal integer string=w461:string)  [unwired: 1 in]
                n215 = Number To Decimal String(number=w460) -> (decimal integer string=w459:string)  [unwired: 1 in]
                n216 = Number To Decimal String(number=w456) -> (decimal integer string=w453:string)  [unwired: 1 in]
                n217 = Close Reference(reference=w468) -> ()  [unwired: 1 in, 1 out]
                n218 = Concatenate Strings(w472, "  Slot ID: " ("字符串"), w461, "  Cycle: " ("字符串"), w459, " Repetition: " ("字符串"), w455, " length: " ("字符串"), w453) -> (w449:string)
                n219 = Bundle By Name(cluster=T5 {"Left Cell String"="", "Child Text"=[], "Child Tag"="", "Item Indent"=0, "Child Only?"=FALSE, "Glyph Index"=0} ("Item"), "Left Cell String"=w449, "Child Text"=string[] [], "Child Tag"=w449, "Item Indent"=1 ("新项缩进"), "Child Only?"=FALSE ("仅作为子项？"), "Glyph Index"=0) -> (w446:T5)
                n220 = Build Array (concatenate)(w444, w446) -> (w445:T4)
                n221 = for {
                  N: w469 -> [_]
                  tunnel: w467 -> [w510]
                  tunnel: w466 -> [w509]
                  tunnel: w465 -> [w508]
                  shift-right: [w504] -> w463
                  shift-left: w464 -> [w507]
                  shift-right: [w482] -> w443
                  shift-left: w445 -> [w480]
                  i -> [w511]
                  n222 = constructor class="TDBSignalProperties"() -> (reference out=w513:refnum<k24>)  [unwired: 3 in, 2 out]
                  n223 = property on="属性节点" class="TDBSignalProperties"(reference=w513, "FDBIndex"=w510, "FECUIndex"=w509, "FFrameIndex"=w508, "FSignalIndex"=w511, "FIsTx"=u8 1) -> (reference out=w506:refnum<k24>)  [unwired: 1 in, 1 out]
                  n224 = invoke on="调用节点" class="TsMasterApi" method="tsdb_get_flexray_db_signal_properties_by_index"(error in=w507, "Avalue"=w506) -> (error out=w504:errorcluster, "Avalue"=w505:refnum<k24>)  [unwired: 2 in, 2 out]
                  n225 = property on="属性节点" class="TDBSignalProperties"(reference=w505) -> (reference out=w503:refnum<k24>, "FDBName"=w501:string, "FFlexRaySignal"=w502:refnum<k24>)  [unwired: 1 in, 1 out]
                  n226 = property on="属性节点" class="TFlexRaySignal"(reference=w502) -> ("FStartBit"=w496:i32, "FLength"=w497:i32, "FFactor"=w498:dbl, "FOffset"=w499:dbl)  [unwired: 1 in, 2 out]
                  n227 = Number To Decimal String(number=w496) -> (decimal integer string=w495:string)  [unwired: 1 in]
                  n228 = Number To Decimal String(number=w498) -> (decimal integer string=w491:string)  [unwired: 1 in]
                  n229 = Number To Decimal String(number=w497) -> (decimal integer string=w493:string)  [unwired: 1 in]
                  n230 = Number To Decimal String(number=w499) -> (decimal integer string=w489:string)  [unwired: 1 in]
                  n231 = Concatenate Strings(w501, "    开始位：" ("字符串"), w495, "    长度：" ("字符串"), w493, "    因子：" ("字符串"), w491, "    偏移量：" ("字符串"), w489) -> (w484:string)
                  n232 = Close Reference(reference=w503) -> ()  [unwired: 1 in, 1 out]
                  n233 = Bundle By Name(cluster=T5 {"Left Cell String"="", "Child Text"=[], "Child Tag"="", "Item Indent"=0, "Child Only?"=FALSE, "Glyph Index"=0} ("Item"), "Left Cell String"=w484, "Child Text"=string[] [], "Child Tag"=w484, "Item Indent"=2 ("新项缩进"), "Child Only?"=TRUE ("仅作为子项？"), "Glyph Index"=0) -> (w481:T5)
                  n234 = Build Array (concatenate)(w480, w481) -> (w482:T4)
                }
              }
            }
            n235 = Close Reference(reference=w415) -> ()  [unwired: 1 in, 1 out]
            n236 = invoke on="flexray database" class="Tree (严格)" method="Edit Tree Items.Add Multiple Items to End"("Items"=w411) -> ()  [unwired: 3 in, 4 out]
          }
        }
      }
      event "transmit": Value Change {
        n237 = event-data() -> ()  [unwired: 1 in, 6 out]
        n238 = case shown="\"CAN\"" "transtab" {
          tunnel: "transmit" -> [_ _ _ _]
          tunnel: [w677 w693 w706 0 ("tsapp_transmit_flexray_async")] -> w668
          frame "CAN" {
            n239 = constructor class="TLIBCANFD"() -> (reference out=w692:refnum<k24>)  [unwired: 3 in, 2 out]
            n240 = Initialize Array(u8 0 ("元素"), 64 ("维数大小")) -> (w681:u8[])
            n241 = Replace Array Subset(array=w681, new element="数据", index=0 ("索引")) -> (w678:u8[])
            n242 = property on="属性节点" class="TLIBCANFD"(reference=w692, "FIdxChn"="CAN通道", "FIdentifier"="CAN ID", "FIsRemote"="是否远程帧", "FIsExt"="是否扩展帧", "FIsFD"="是否CAN FD", "FIsBRS"="是否BRS", "FDLC"="DLC", "FData"=w678) -> (reference out=w691:refnum<k24>)  [unwired: 1 in, 1 out]
            n243 = invoke on="调用节点" class="TsMasterApi" method="tsapp_transmit_canfd_async"("ACANFD"=w691) -> ("tsapp_transmit_canfd_async"=w677:i32)  [unwired: 3 in, 3 out]
          }
          frame "LIN" {
            n244 = constructor class="TLIBLIN"() -> (reference out=w705:refnum<k24>)  [unwired: 3 in, 2 out]
            n245 = Initialize Array(u8 0 ("元素"), 8 ("维数大小")) -> (w697:u8[])
            n246 = Replace Array Subset(array=w697, new element="数据", index=0 ("索引")) -> (w694:u8[])
            n247 = property on="属性节点" class="TLIBLIN"(reference=w705, "FIdxChn"="LIN通道", "FIdentifier"="LIN ID", "FIsTx"="是否包含数据", "FDLC"="长度", "FData"=w694) -> (reference out=w704:refnum<k24>)  [unwired: 1 in, 1 out]
            n248 = invoke on="调用节点" class="TsMasterApi" method="tsapp_transmit_lin_async"("ALIN"=w704) -> ("tsapp_transmit_lin_async"=w693:i32)  [unwired: 3 in, 3 out]
          }
          frame "flexray" {
            n249 = constructor class="TLIBFlexray"() -> (reference out=w719:refnum<k24>)  [unwired: 3 in, 2 out]
            n250 = Initialize Array(u8 0 ("元素"), 254 ("维数大小")) -> (w715:u8[])
            n251 = Replace Array Subset(array=w715, new element="数据 2", index=0 ("索引")) -> (w712:u8[])
            n252 = property on="属性节点" class="TLIBFlexray"(reference=w719, "FIdxChn"="flexray通道", "FSlotId"="SlotId", "FCycleNumber"="CycleNumber", "FPayloadLength"="负载长度", "FData"=w712, "FChannelMask"=u8 1, "FActualPayloadLength"="负载长度") -> (reference out=w718:refnum<k24>)  [unwired: 1 in, 1 out]
            n253 = invoke on="调用节点" class="TsMasterApi" method="tsapp_transmit_flexray_async"("AFlexray"=w718) -> ("tsapp_transmit_flexray_async"=w706:i32)  [unwired: 3 in, 3 out]
          }
          frame Default {
          }
        }
        n254 = Not Equal To 0?(x=w668) -> (x != 0?=w669:bool)
        n255 = case shown="真" w669 {
          tunnel: w668 -> [_ w672]
          frame False {
          }
          frame True {
            n256 = Number To Decimal String(number=w672) -> (decimal integer string=w675:string)  [unwired: 1 in]
            n257 = Concatenate Strings("\r\n", "发送失败：" ("字符串"), w675) -> (w673:string)
            n258 = invoke on="log" class="Str" method="Append String"("string"=w673) -> ()  [unwired: 3 in, 4 out]
          }
        }
      }
    }
    n259 = local read "使能CAN通道数量"() -> (w25:i32)
    n260 = local read "使能LIN通道数量"() -> (w24:i32)
    n261 = property on="报文信息" class="MCListbox (严格)"() -> ("ItemNames"=w23:string[][])  [unwired: 2 in, 2 out]
    n262 = for {
      N: w25 -> [_]
      shift-right: [w145] -> w22
      shift-left: w23 -> [w146]
      i -> [w147]
      n263 = invoke on="调用节点" class="TsMasterApi" method="tsfifo_read_canfd_buffer_frame_count"("AChn"=w147, "ACount"=0) -> ("ACount"=w148:i32)  [unwired: 3 in, 4 out]
      n264 = for {
        N: w148 -> [_]
        tunnel: w147 -> [w152]
        shift-right: [w150] -> w145
        shift-left: w146 -> [w151]
        w153 = u8 1 items=["ONLY_RX_MESSAGES", "TX_RX_MESSAGES"] ("ARxTx")
        n265 = constructor class="TLIBCANFD"() -> (reference out=w155:refnum<k24>)  [unwired: 3 in, 2 out]
        n266 = invoke on="调用节点" class="TsMasterApi" method="tsfifo_receive_canfd_message"("ACANMsg"=w155, "ATimeoutMs"=100, "AChn"=w152, "ARxTx"=w153) -> ("tsfifo_receive_canfd_message"=w157:bool, "ACANMsg"=w156:refnum<k24>)  [unwired: 3 in, 5 out]
        n267 = case shown="真" w157 {
          tunnel: w156 -> [w158 w206]
          tunnel: w151 -> [w159 w162]
          tunnel: [w159 w161] -> w150
          frame False {
            n268 = Close Reference(reference=w158) -> ()  [unwired: 1 in, 1 out]
          }
          frame True {
            w189 = ""
            n269 = property on="属性节点" class="TLIBCANFD"(reference=w206) -> (reference out=w160:refnum<k24>, "FTimeUS"=w205:u64, "FIdxChn"=w167:u8, "FIdentifier"=w197:i32, "FIsTx"=w195:bool, "FIsRemote"=w191:bool, "FIsExt"=w164:bool, "FIsFD"=w187:bool, "FIsBRS"=w185:bool, "FIsESI"=w183:bool, "FDLC"=w174:u8, "FData"=w172:u8[])  [unwired: 1 in, 1 out]
            n270 = Increment(x=w167) -> (x+1=w168:u8)
            n271 = call "CANDLC.vi"("DLC"=w174) -> ("length"=w173:u8)
            n272 = Number To Decimal String(number=w168) -> (decimal integer string=w200:string)  [unwired: 1 in]
            n273 = Divide(x=w205, y=u64 1000) -> (x/y=w203:dbl)
            n274 = Select(t="Tx", s=w195, f="Rx") -> (s? t:f=w192:string)
            n275 = Select(t=i16 8, s=w164, f=i16 3 ("精度(6)")) -> (s? t:f=w166:i16)
            n276 = for {
              N: w173 -> [_]
              tunnel: w172 -> [w212] mode=indexing
              shift-right: [w207] -> w170
              shift-left: "" -> [w210]
              n277 = Number To Hexadecimal String(1:i16 2 ("宽度(-)"), 2:w212) -> (0:w209:string)
              n278 = call <vilib>:"Space Constant.vi"() -> ("String"=w208:string)
              n279 = Concatenate Strings(w210, w209, w208) -> (w207:string)
            }
            n280 = Number To Decimal String(number=w173) -> (decimal integer string=w175:string)  [unwired: 1 in]
            n281 = Number To Fractional String(number=w203, precision (6)=i16 3 ("精度(6)")) -> (F-format string=w201:string)  [unwired: 2 in]
            n282 = Concatenate Strings("CAN" ("字符串"), w200) -> (w198:string)
            n283 = Number To Hexadecimal String(1:w166, 2:w197) -> (0:w196:string)
            n284 = Select(t="RTR ", s=w191, f=w189) -> (s? t:f=w180:string)
            n285 = Select(t="FD ", s=w187, f=w189) -> (s? t:f=w179:string)
            n286 = Select(t="ESI ", s=w183, f=w189) -> (s? t:f=w177:string)
            n287 = Select(t="EXT ", s=w164, f=w189) -> (s? t:f=w181:string)
            n288 = Select(t="BRS ", s=w185, f=w189) -> (s? t:f=w178:string)
            n289 = Concatenate Strings(w180, w181, w179, w178, w177) -> (w176:string)
            n290 = Close Reference(reference=w160) -> ()  [unwired: 1 in, 1 out]
            n291 = Build Array(w201, w198, w196, w192, w176, w175, w170) -> (w169:string[])
            n292 = call "message.vi"("itemlist"=w162, "item"=w169) -> ("itemlistout"=w161:string[][])
          }
        }
      }
    }
    n293 = property on="报文信息" class="MCListbox (严格)"("ItemNames"=w22) -> (error out=w16:errorcluster)  [unwired: 2 in, 1 out]
    n294 = property on="报文信息" class="MCListbox (严格)"(error in=w16) -> ("ItemNames"=w21:string[][])  [unwired: 1 in, 2 out]
    n295 = for {
      N: w24 -> [_]
      shift-right: [w96] -> w20
      shift-left: w21 -> [w97]
      i -> [w98]
      n296 = invoke on="调用节点" class="TsMasterApi" method="tsfifo_read_lin_buffer_frame_count"("AChn"=w98, "ACount"=0) -> ("ACount"=w99:i32)  [unwired: 3 in, 4 out]
      n297 = for {
        N: w99 -> [_]
        tunnel: w98 -> [w103]
        shift-right: [w101] -> w96
        shift-left: w97 -> [w102]
        w104 = u8 1 items=["ONLY_RX_MESSAGES", "TX_RX_MESSAGES"] ("ARxTx")
        n298 = constructor class="TLIBLIN"() -> (reference out=w106:refnum<k24>)  [unwired: 3 in, 2 out]
        n299 = invoke on="调用节点" class="TsMasterApi" method="tsfifo_receive_lin_message"("ALINMsg"=w106, "ATimeoutMs"=100, "AChn"=w103, "ATxRx"=w104) -> ("tsfifo_receive_lin_message"=w108:bool, "ALINMsg"=w107:refnum<k24>)  [unwired: 3 in, 5 out]
        n300 = case shown="真" w108 {
          tunnel: w107 -> [w109 w138]
          tunnel: w102 -> [w110 w113]
          tunnel: [w110 w112] -> w101
          frame False {
            n301 = Close Reference(reference=w109) -> ()  [unwired: 1 in, 1 out]
          }
          frame True {
            n302 = property on="属性节点" class="TLIBLIN"(reference=w138) -> (reference out=w111:refnum<k24>, "FTimeUS"=w137:u64, "FIdxChn"=w118:u8, "FIdentifier"=w129:u8, "FIsTx"=w127:bool, "FDLC"=w115:u8, "FData"=w114:u8[])  [unwired: 1 in, 1 out]
            n303 = Increment(x=w118) -> (x+1=w119:u8)
            n304 = Number To Decimal String(number=w119) -> (decimal integer string=w132:string)  [unwired: 1 in]
            n305 = Divide(x=w137, y=u64 1000) -> (x/y=w135:dbl)
            n306 = Select(t="Tx", s=w127, f="Rx") -> (s? t:f=w124:string)
            n307 = for {
              N: w115 -> [_]
              shift-right: [w140] -> w121
              shift-left: "" -> [w143]
              tunnel: w114 -> [w139] mode=indexing
              n308 = Number To Hexadecimal String(1:i16 2 ("宽度(-)"), 2:w139) -> (0:w142:string)
              n309 = call <vilib>:"Space Constant.vi"() -> ("String"=w141:string)
              n310 = Concatenate Strings(w143, w142, w141) -> (w140:string)
            }
            n311 = Number To Decimal String(number=w115) -> (decimal integer string=w123:string)  [unwired: 1 in]
            n312 = Number To Fractional String(number=w135, precision (6)=i16 3 ("精度(6)")) -> (F-format string=w133:string)  [unwired: 2 in]
            n313 = Concatenate Strings("LIN" ("字符串"), w132) -> (w130:string)
            n314 = Number To Hexadecimal String(1:i16 2 ("宽度(-)"), 2:w129) -> (0:w128:string)
            n315 = Close Reference(reference=w111) -> ()  [unwired: 1 in, 1 out]
            n316 = Build Array(w133, w130, w128, w124, "" ("元素"), w123, w121) -> (w120:string[])
            n317 = call "message.vi"("itemlist"=w113, "item"=w120) -> ("itemlistout"=w112:string[][])
          }
        }
      }
    }
    n318 = property on="报文信息" class="MCListbox (严格)"("ItemNames"=w20) -> (error out=w15:errorcluster)  [unwired: 2 in, 1 out]
    n319 = property on="报文信息" class="MCListbox (严格)"(error in=w15) -> ("ItemNames"=w18:string[][])  [unwired: 1 in, 2 out]
    n320 = for {
      N: w17 -> [_]
      shift-right: [w35] -> w19
      shift-left: w18 -> [w36]
      i -> [w30]
      w32 = 1000 ("y")
      n321 = invoke on="调用节点" class="TsMasterApi" method="tsfifo_read_flexray_buffer_frame_count"("channel"=w30, "ACount"=0) -> (error out=w29:errorcluster, "ACount"=w33:i32)  [unwired: 3 in, 3 out]
      n322 = Greater?(x=w33, y=w32) -> (0:w34:bool)
      n323 = Select(t=w32, s=w34, f=w33) -> (s? t:f=w31:i32)
      n324 = for {
        N: w31 -> [_]
        tunnel: w30 -> [w44]
        shift-right: [w46] -> w35
        shift-left: w36 -> [w47]
        shift-right: [w38] -> w28
        shift-left: w29 -> [w39]
        w45 = u8 1 items=["ONLY_RX_MESSAGES", "TX_RX_MESSAGES"] ("ARxTx")
        n325 = constructor class="TLIBFlexray"() -> (reference out=w40:refnum<k24>)  [unwired: 3 in, 2 out]
        n326 = invoke on="调用节点" class="TsMasterApi" method="tsfifo_receive_flexray_message"(error in=w39, "AFlexrayMsg"=w40, "ATimeoutMs"=100, "AChn"=w44, "ATxRx"=w45) -> (error out=w38:errorcluster, "tsfifo_receive_flexray_message"=w42:bool, "AFlexrayMsg"=w41:refnum<k24>)  [unwired: 2 in, 4 out]
        n327 = case shown="真" w42 {
          tunnel: w47 -> [w49 w73]
          tunnel: [w49 w72] -> w46
          tunnel: w41 -> [w48 w51]
          frame False {
            n328 = Close Reference(reference=w48) -> ()  [unwired: 1 in, 1 out]
          }
          frame True {
            w59 = ""
            n329 = property on="属性节点" class="TLIBFlexray" props=["FTimeUs", "FIdxChn", "FSlotId", "FCycleNumber", "FDir", "FFrameFlags", "FActualPayloadLength", "FData"](reference=w51) -> (reference out=w52:refnum<k24>, "FTimeUs"=w71:u64, "FIdxChn"=w74:u8, "FSlotId"=w53:u16, "FDir"=w69:u8, "FFrameFlags"=w66:u32, "FActualPayloadLength"=w67:u8, "FData"=w68:u8[])  [unwired: 1 in, 2 out]
            n330 = Increment(x=w74) -> (x+1=w75:u8)
            n331 = Greater Than 0?(x=w69) -> (x > 0?=w70:bool)
            n332 = Divide(x=w71, y=u64 1000) -> (x/y=w88:dbl)
            n333 = Number To Decimal String(number=w75) -> (decimal integer string=w85:string)  [unwired: 1 in]
            n334 = Select(t="Tx", s=w70, f="Rx") -> (s? t:f=w80:string)
            n335 = for {
              N: w67 -> [_]
              shift-right: [w91] -> w77
              shift-left: "" -> [w94]
              tunnel: w68 -> [w90] mode=indexing
              n336 = Number To Hexadecimal String(1:i16 2 ("宽度(-)"), 2:w90) -> (0:w93:string)
              n337 = call <vilib>:"Space Constant.vi"() -> ("String"=w92:string)
              n338 = Concatenate Strings(w94, w93, w92) -> (w91:string)
            }
            n339 = Number To Decimal String(number=w67) -> (decimal integer string=w79:string)  [unwired: 1 in]
            n340 = Number To Fractional String(number=w88, precision (6)=i16 3 ("精度(6)")) -> (F-format string=w86:string)  [unwired: 2 in]
            n341 = Concatenate Strings("Flexray" ("字符串"), w85) -> (w83:string)
            n342 = And(x=w66, y=u32 1) -> (x .and. y?=w63:u32)
            n343 = And(x=w66, y=u32 8) -> (x .and. y?=w62:u32)
            n344 = Number To Decimal String(number=w53) -> (decimal integer string=w50:string)  [unwired: 1 in]
            n345 = Close Reference(reference=w52) -> ()  [unwired: 1 in, 1 out]
            n346 = Greater Than 0?(x=w63) -> (x > 0?=w61:bool)
            n347 = Greater Than 0?(x=w62) -> (x > 0?=w60:bool)
            n348 = Select(t="NULL ", s=w61, f=w59) -> (s? t:f=w56:string)
            n349 = Select(t="StartUP", s=w60, f=w59) -> (s? t:f=w55:string)
            n350 = Concatenate Strings(w56, w55) -> (w54:string)
            n351 = Build Array(w86, w83, w50, w80, w54, w79, w77) -> (w76:string[])
            n352 = call "message.vi"("itemlist"=w73, "item"=w76) -> ("itemlistout"=w72:string[][])
          }
        }
      }
      n353 = invoke on="调用节点" class="TsMasterApi" method="tsfifo_clear_flexray_receive_buffers"(error in=w28, "channel"=w30) -> ()  [unwired: 2 in, 4 out]
    }
    n354 = property on="报文信息" class="MCListbox (严格)"("ItemNames"=w19) -> ()  [unwired: 2 in, 2 out]
  }
  n355 = disable-structure shown="禁用" {
    frame Disabled {
      n356 = invoke on="调用节点" class="TsMasterApi" method="tscom_can_rbs_activate_all_networks"("AEnable"=TRUE, "AIncludingChildren"=FALSE) -> (error out=w729:errorcluster)  [unwired: 3 in, 4 out]
      n357 = invoke on="调用节点" class="TsMasterApi" method="tscom_can_rbs_activate_node_by_name"(error in=w729, "AIdxChn"=0, "AEnable"=TRUE, "ANetworkName"="CAN_FD_Powertrain", "NodeName"="Engine", "AIncludingChildren"=TRUE) -> (error out=w721:errorcluster)  [unwired: 2 in, 7 out]
      n358 = invoke on="调用节点" class="TsMasterApi" method="tscom_can_rbs_start"(error in=w721) -> (error out=w723:errorcluster)  [unwired: 2 in, 2 out]
      n359 = while {
        shift-right: [w735] -> w722
        shift-left: w723 -> [w738]
        stop <- "停止" stop-if-true
        n360 = invoke on="调用节点" class="TsMasterApi" method="tscom_can_rbs_get_signal_value_by_address"(error in=w738, "ASymboladdress"="0/CAN_FD_Powertrain/Engine/Ignition_Info/StarterKey", "AValue"=0.0) -> (error out=w736:errorcluster)  [unwired: 2 in, 4 out]
        n361 = invoke on="调用节点" class="TsMasterApi" method="tscom_can_rbs_set_signal_value_by_address"(error in=w736, "ASymboladdress"="0/CAN_FD_Powertrain/Engine/Test_Message_CAN_FD/Test_Signal_Byte_00") -> (error out=w735:errorcluster)  [unwired: 3 in, 4 out]
        n362 = Wait (ms)(milliseconds to wait=u32 100 ("等待时间（毫秒）")) -> ()  [unwired: 1 out]
      }
      n363 = invoke on="调用节点" class="TsMasterApi" method="tscom_can_rbs_stop"(error in=w722) -> ()  [unwired: 2 in, 3 out]
    }
    frame Enabled {
    }
  }
